vi "Autonomous Independent.vi"   [LabVIEW 2017]
doc: "This VI is called when autonomous begins, and will automatically be terminated when autonomous ends. You can carry out timed or sensor driven robot movement independently without needing to return to the caller."
uses:
  <vilib>/Rock Robotics/WPI/Solenoid/WPI_SolenoidValue.ctl
  <vilib>/Rock Robotics/WPI/ThirdParty/Phoenix-LabVIEW/Motor Controller/Controls/CTRE_Phoenix_MotorControl_ControlMode.ctl
  <vilib>/Rock Robotics/Network Tables/NT Read Number.vi
  <vilib>/Rock Robotics/WPI/Solenoid/WPI_SolenoidSetEnum.vi
  <vilib>/Rock Robotics/Network Tables/NT Write String.vi
panel:
  # "Be sure to right-click and choose Data Operations>>Make Current Value default if you want to save the array values with the VI"
types:
  T1 = enum16{"do_nothing", "cross_baseline_short", "cross_baseline_long", "hot_from_middle", "if_hot_2_cube_else_1_cube", "if_hot_1_cube_else_1_cube", "exchange_from_middle", "forward_switch_if_hot", "exchange_from_outside", "if_hot_2_cube_else_baseline", "if_hot_3_cube_else_baseline", "exchange_and_hot_switch", "hot_from_middle_diagonal", "yet to be named", "If_hot_1_else_baseline", "hot_2_from_middle", ""}
  T2 = typedef "WPI_SolenoidDevRef.ctl" = cluster{"DevStatus":errorcluster, "Pneumatics Control Module":u8, "Forward Solenoid Channel":T3, "Reverse Solenoid Channel":T3}
  T3 = typedef "WPI_SolenoidChannel.ctl" = enum8{"Solenoid 0", "Solenoid 1", "Solenoid 2", "Solenoid 3", "Solenoid 4", "Solenoid 5", "Solenoid 6", "Solenoid 7", "Invalid"}
  T4 = typedef "WPI_SolenoidValue.ctl" = enum16{"Off", "On", "Forward", "Reverse"}
  T5 = typedef "WPI_MotorControlDeviceRef.ctl" = cluster{"DeviceStatus":errorcluster, "Type":T6, "PWM":cluster{"PWM Channel":T7, "DeadBand":T8}, "CAN":cluster{"Device Number":u8, "SetOutput VI Ref":variant, "GetOutput VI Ref":variant, "Enable VI Ref":variant, "Disable VI Ref":variant, "Data":variant}, "Invert":bool, "DIO PWM":cluster{"PWM \"Enable\" Channel":T7, "DIOChannel":T9, "PWM Rate":dbl}}
  T6 = typedef "WPI_MotorControlType.ctl" = enum16{"PWM", "CAN", "DIO PWM"}
  T7 = typedef "FPGA_DIOPWMChannel.ctl" = enum8{"PWM 0", "PWM 1", "PWM 2", "PWM 3", "PWM 4", "PWM 5", "PWM 6", "PWM 7", "PWM 8", "PWM 9", "PWM MXP 0", "PWM MXP 1", "PWM MXP 2", "PWM MXP 3", "PWM MXP 4", "PWM MXP 5", "PWM MXP 6", "PWM MXP 7", "PWM MXP 8", "PWM MXP 9", "Invalid"}
  T8 = typedef "WPI_PWMDeadband.ctl" = cluster{"Name":string, "maxPositivePwm":i32, "minPositivePwm":i32, "centerPwm":i32, "maxNegativePwm":i32, "minNegativePwm":i32, "angularRange":u16}
  T9 = typedef "FPGA_DIOChannel.ctl" = enum8{"DIO 0", "DIO 1", "DIO 2", "DIO 3", "DIO 4", "DIO 5", "DIO 6", "DIO 7", "DIO 8", "DIO 9", "DIO MXP 0", "DIO MXP 1", "DIO MXP 2", "DIO MXP 3", "DIO MXP 4", "DIO MXP 5", "DIO MXP 6", "DIO MXP 7", "DIO MXP 8", "DIO MXP 9", "DIO MXP 10", "DIO MXP 11", "DIO MXP 12", "DIO MXP 13", "DIO MXP 14", "DIO MXP 15", "SPI Port CS1", "SPI Port CS2", "SPI Port CS3", "SPI Port MISO", "SPI Port MOSI", "Invalid"}
  T10 = typedef "CTRE_Phoenix_MotorControl_ControlMode.ctl" = u16
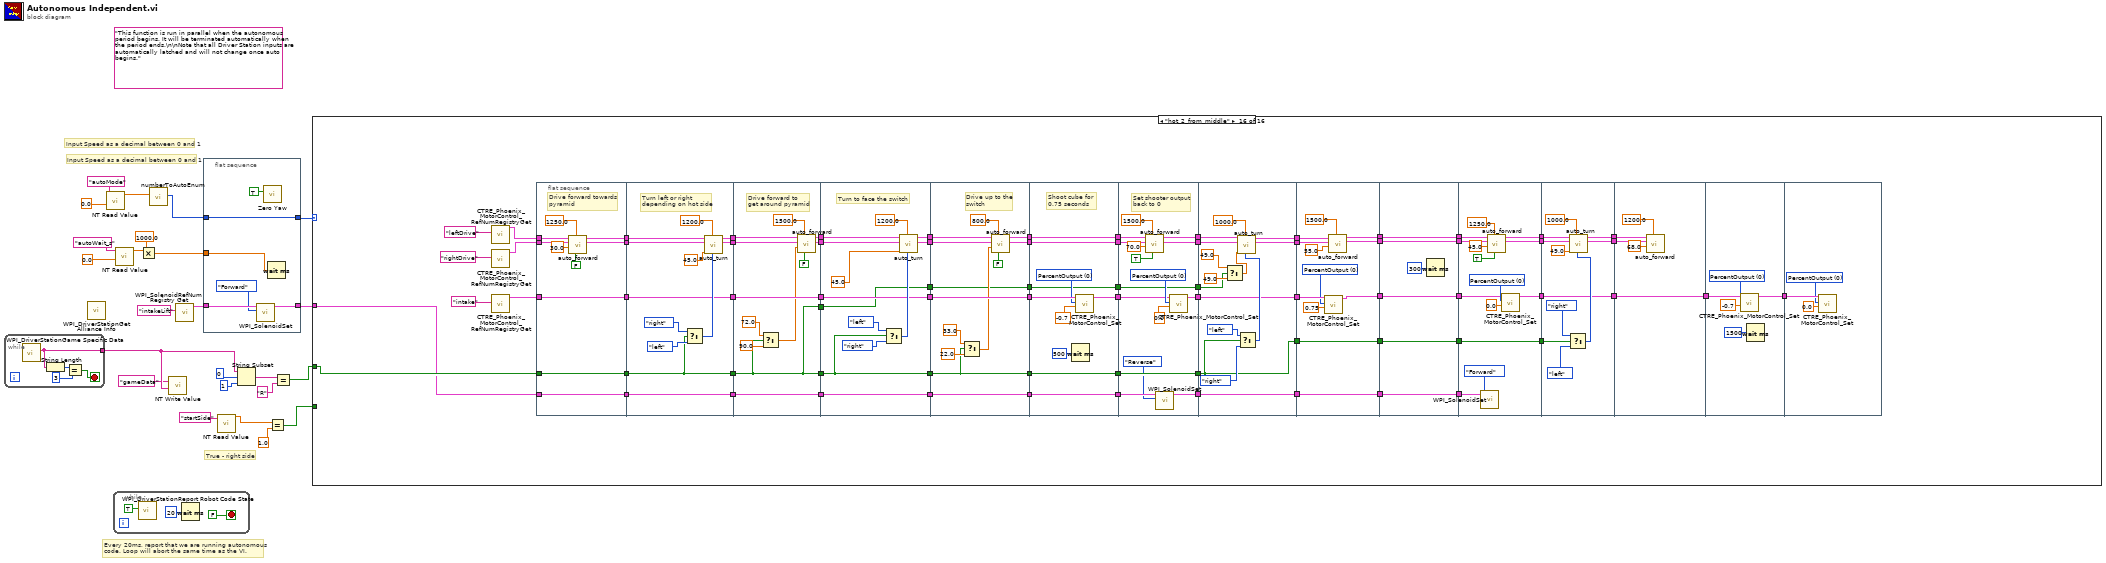
[diagram p0: block diagram]
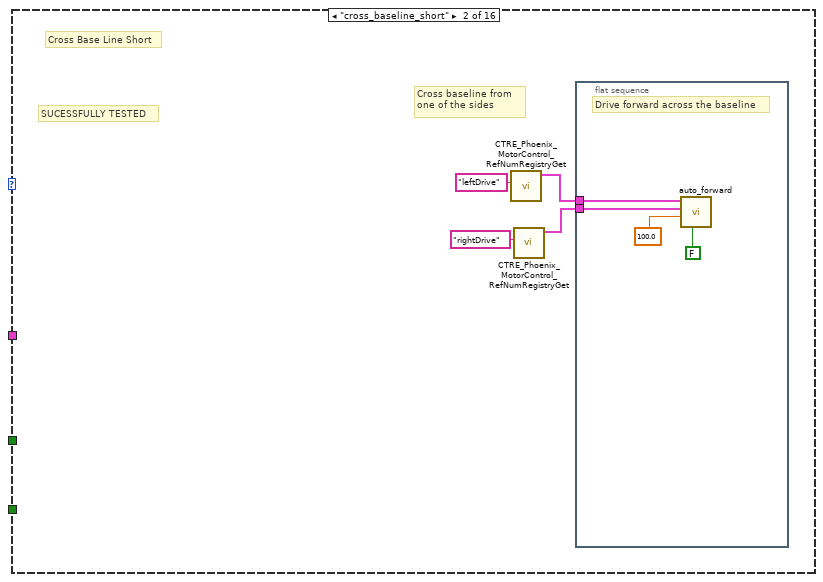
[diagram p3: hidden frame]
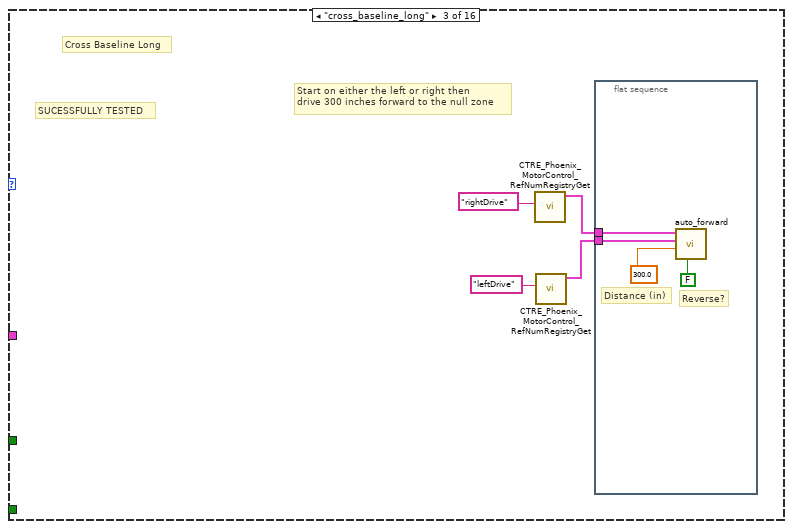
[diagram p4: hidden frame]
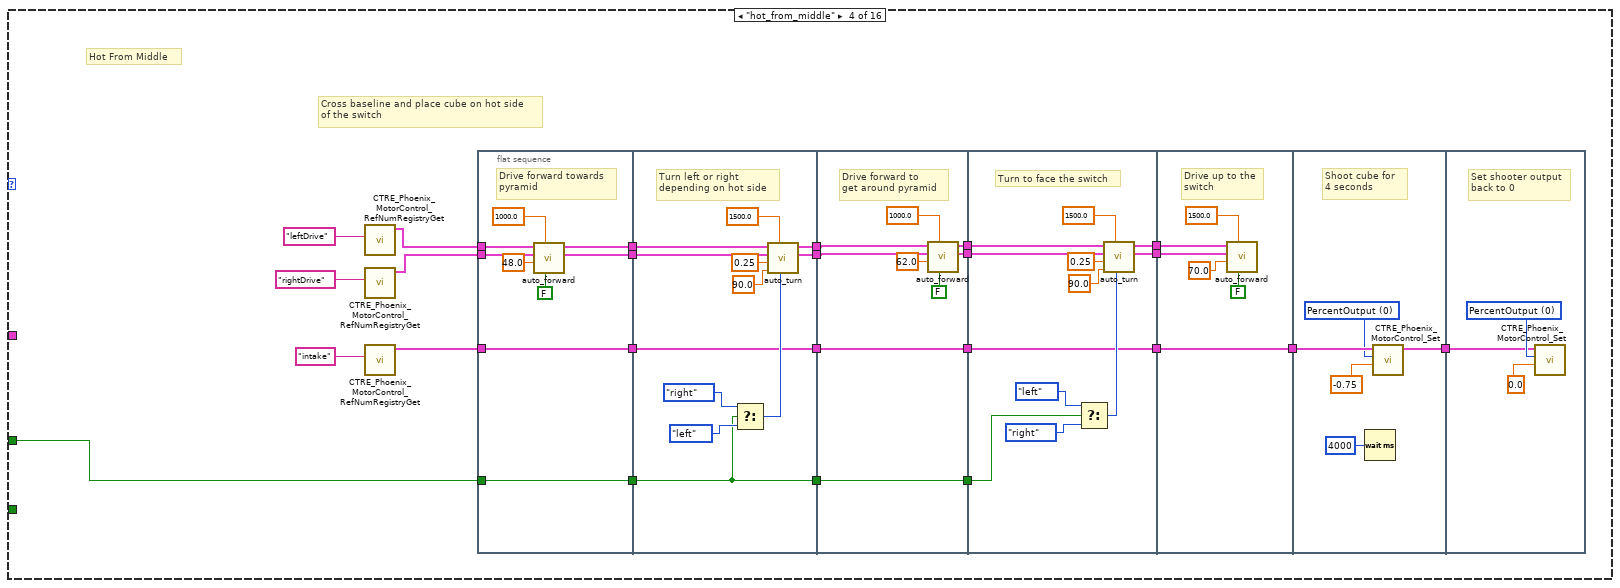
[diagram p5: hidden frame]
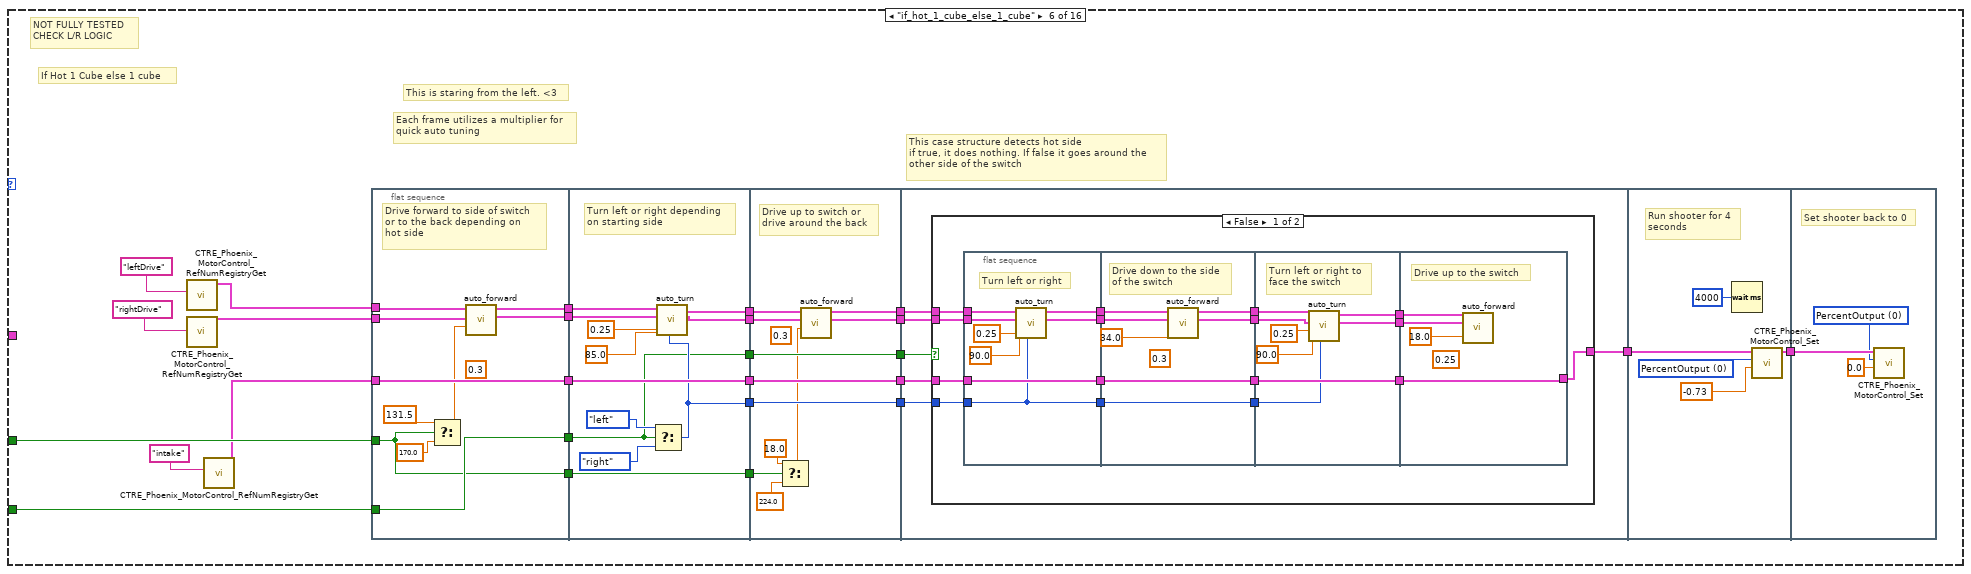
[diagram p7: hidden frame]
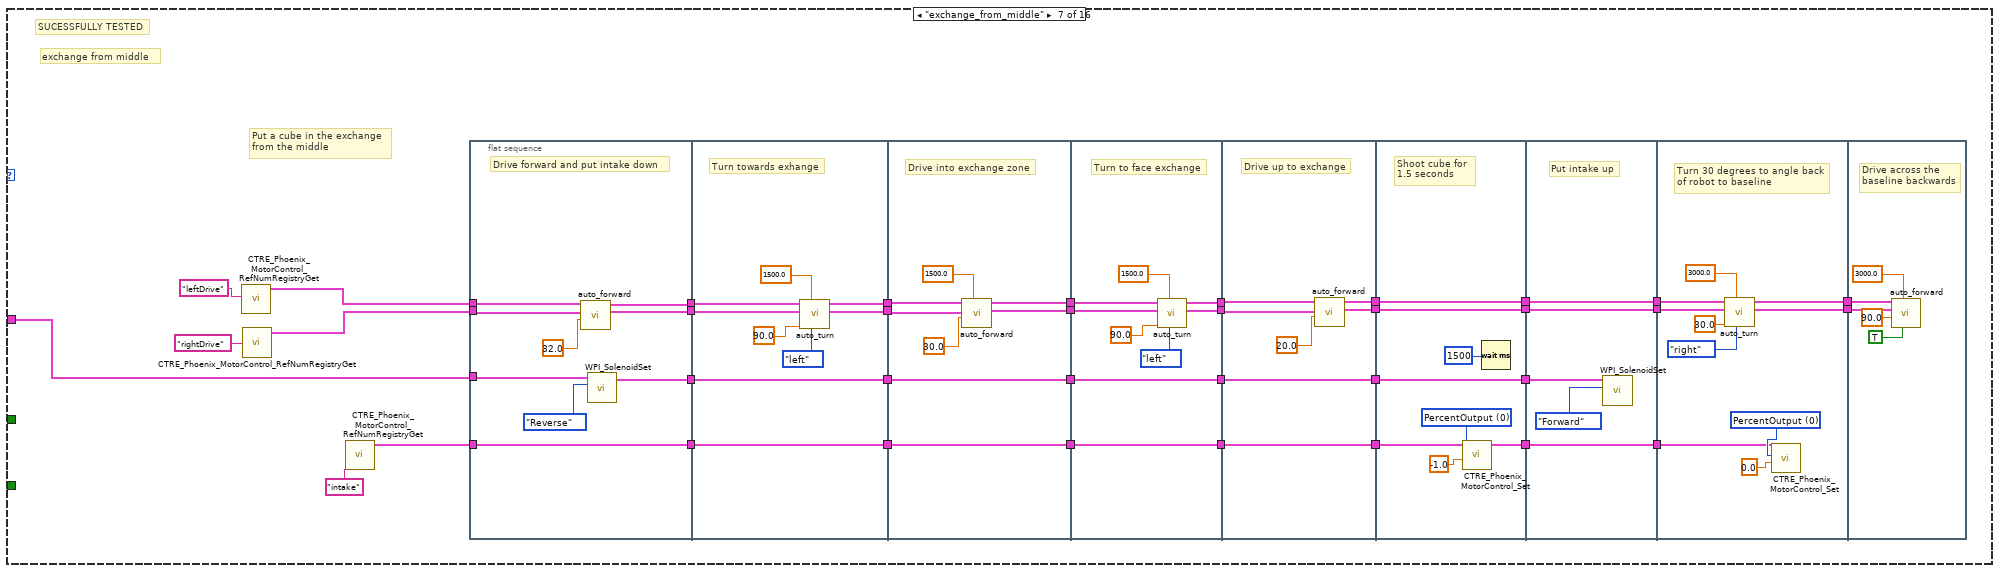
[diagram p9: hidden frame]
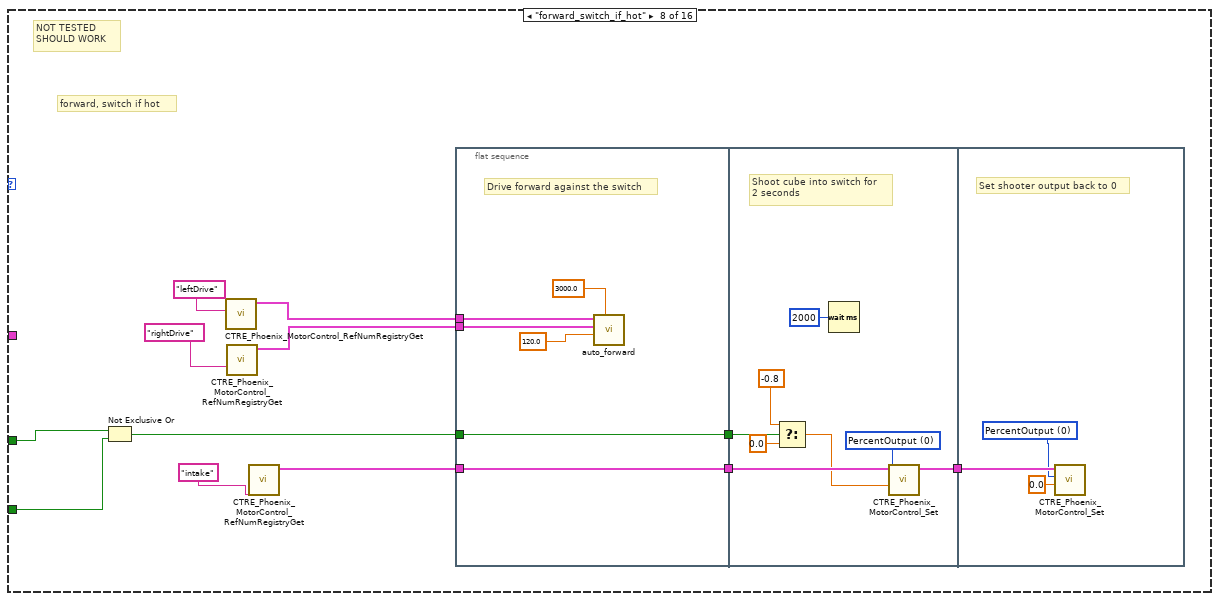
[diagram p10: hidden frame]
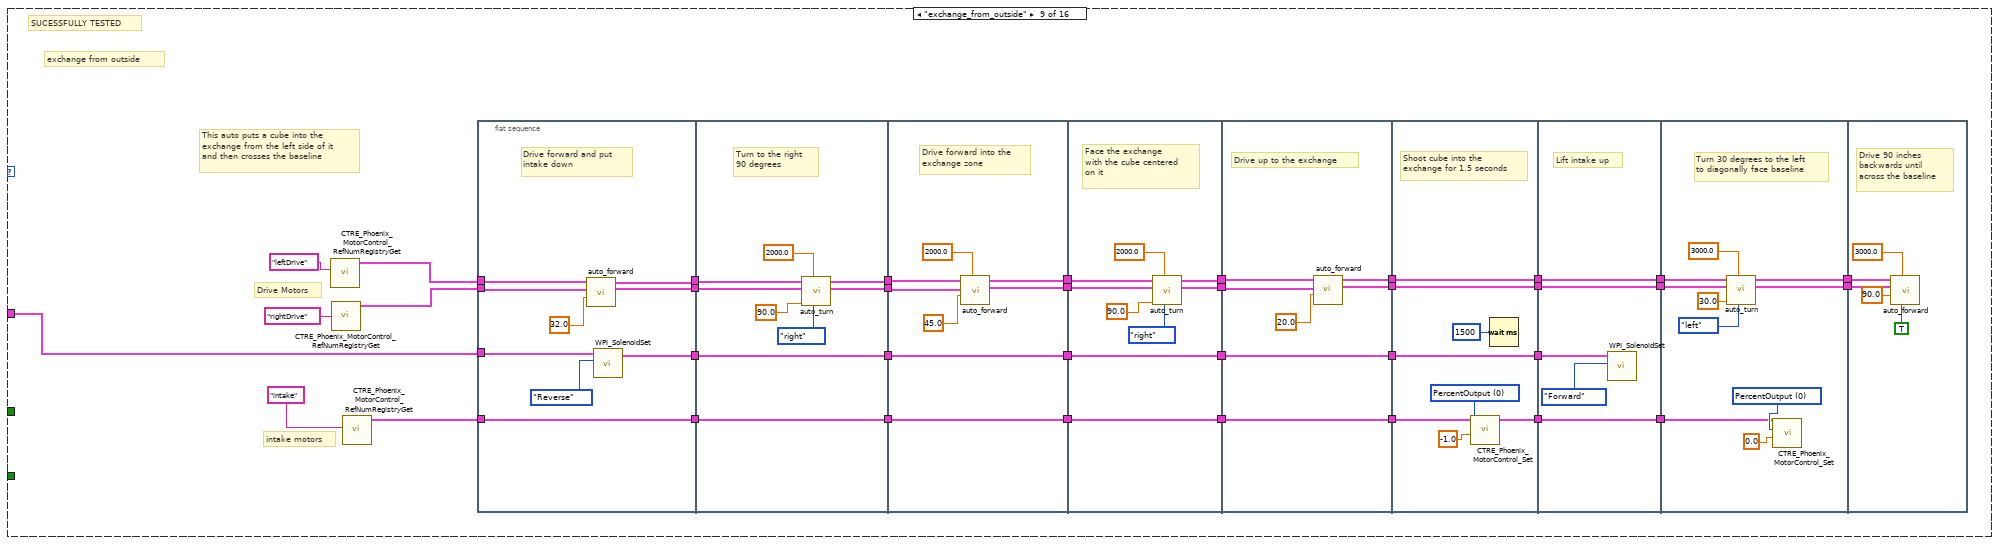
[diagram p11: hidden frame]
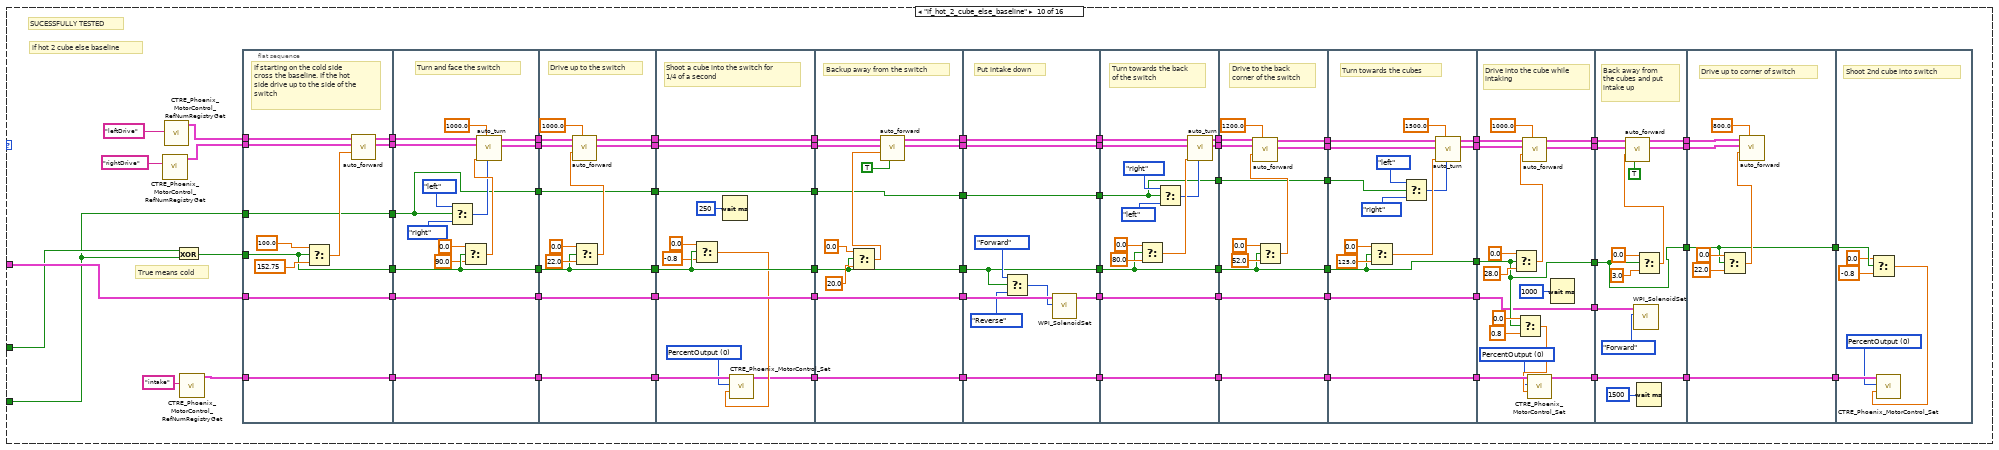
[diagram p12: hidden frame]
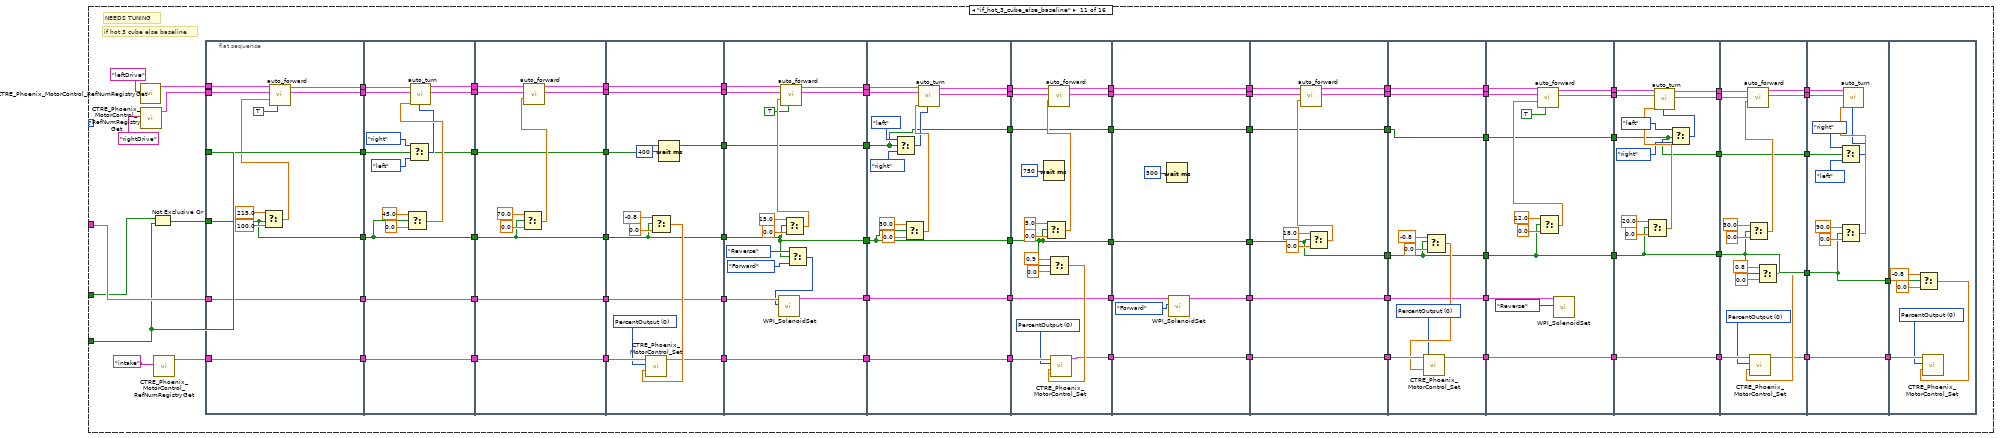
[diagram p13: hidden frame]
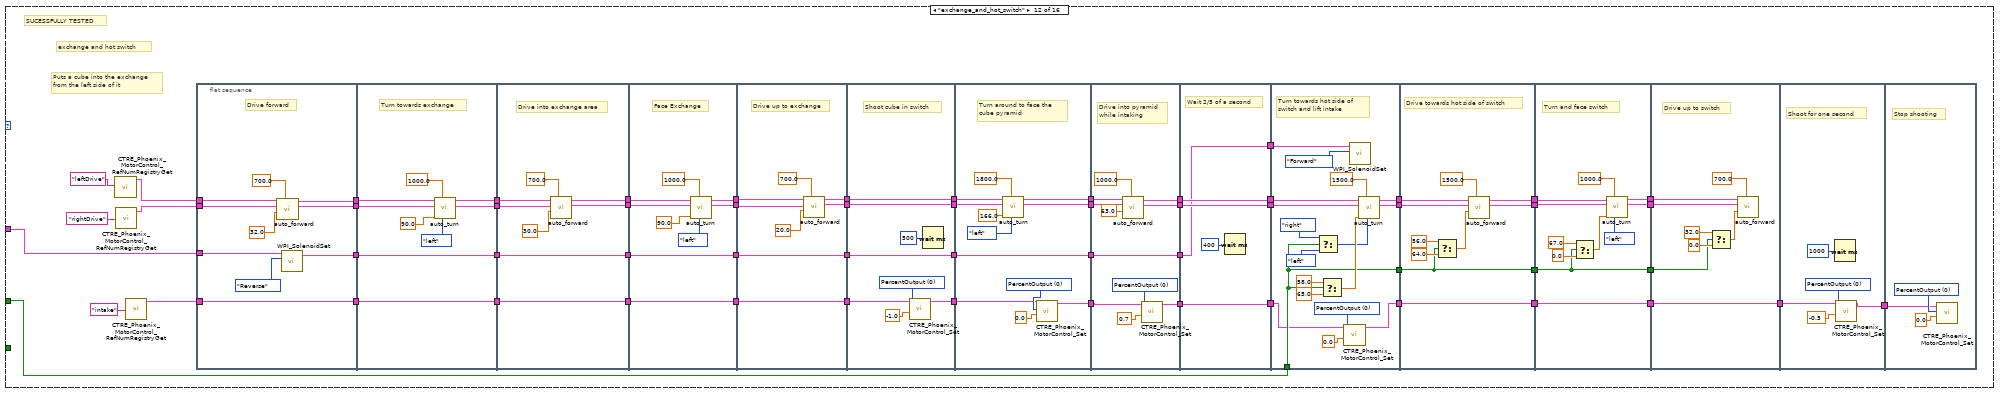
[diagram p14: hidden frame]
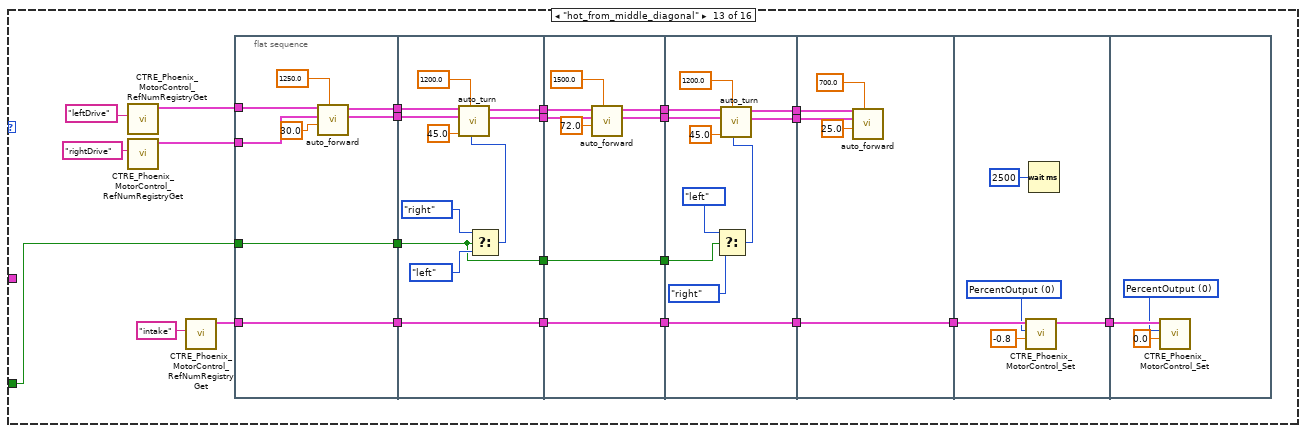
[diagram p15: hidden frame]
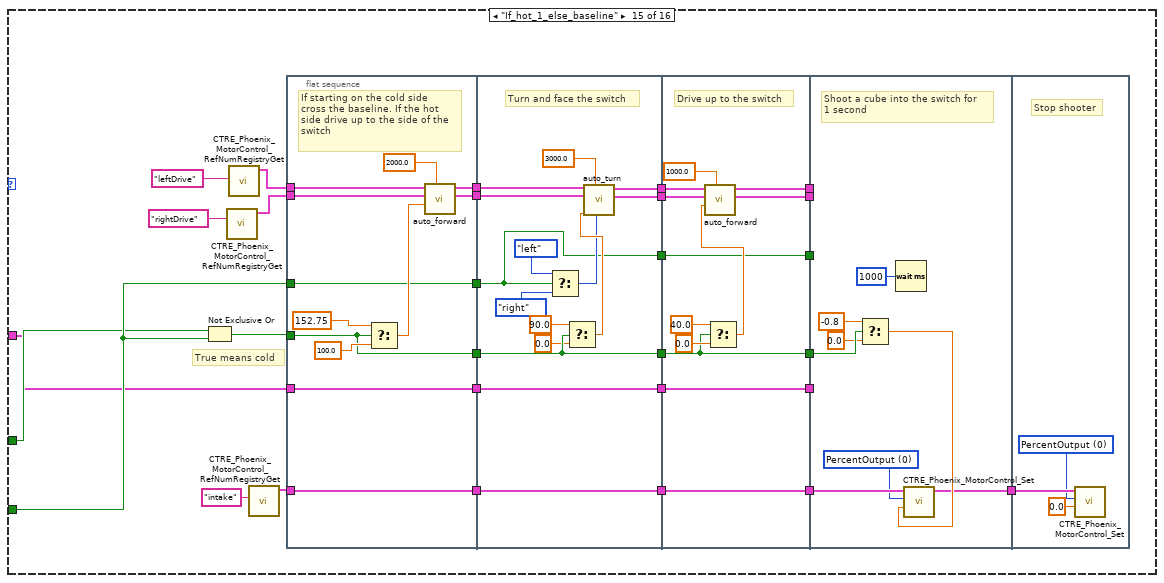
[diagram p17: hidden frame]
diagram:
  (unwired) "This function is run in parallel when the autonomous period begins. It will be terminated automatically when the period ends.\n\nNote that all Driver Station inputs are automatically latched and will not change once auto begins."
  # "True - right side"
  # "Input Speed as a decimal between 0 and 1"
  # "Input Speed as a decimal between 0 and 1"
  # "Every 20ms, report that we are running autonomous\ncode. Loop will abort the same time as the VI."
  n1 = while {
    tunnel: [w28] -> w2
    stop <- w25 stop-if-true
    n2 = call <vilib>:"WPI_DriverStationGame Specific Data.vi"() -> ("Game Specific Data"=w28:string)  [unwired: 11 in]
    n3 = String Length(string=w28) -> (length=w27:i32)
    n4 = Equal?(x=w27, y=3) -> (x = y?=w25:bool)
  }
  n5 = call <vilib>:"WPI_DriverStationGet Alliance Info.vi"() -> ()  [unwired: 12 out]
  n6 = call-poly <vilib>:"NT Read Value.vi"("Default Value"=0.0, "Name"="autoMode") -> ("Numeric"=w5:dbl)  [unwired: 8 in, 1 out]
  n7 = while {
    stop <- FALSE stop-if-true
    n8 = call <vilib>:"WPI_DriverStationReport Robot Code State.vi"("Autonomous"=TRUE) -> ()  [unwired: 10 in, 1 out]
    n9 = Wait (ms)(milliseconds to wait=u32 20) -> ()  [unwired: 1 out]
  }
  n10 = call-poly <vilib>:"NT Read Value.vi"("Default Value"=0.0, "Name"="autoWait_s") -> ("Numeric"=w23:dbl)  [unwired: 8 in, 1 out]
  n11 = Multiply(x=w23, y=1000.0) -> (x*y=w17:dbl)
  n12 = call "numberToAutoEnum.vi"("inNumber"=w5) -> ("outEnum"=w3:T1)  [unwired: 10 in]
  n13 = call-poly <vilib>:"NT Write Value.vi"("String"=w2, "Name"="gameData") -> ()  [unwired: 9 in, 1 out]
  n14 = call <vilib>:"WPI_SolenoidRefNum Registry Get.vi"("refnum name"="intakeLift") -> ("SolenoidDevRef"=w15:T2)  [unwired: 9 in, 1 out]
  n15 = flat-sequence {
    tunnel: w17 -> [w37]
    tunnel: w15 -> [w36]
    tunnel: [w34] -> w14
    tunnel: [w32] -> w4
    tunnel: w3 -> [w32]
    frame #0 {
      n16 = call-poly <vilib>:"WPI_SolenoidSet.vi"("Value"=WPI_SolenoidValue."Forward", "SolenoidDevRef"=w36) -> ("SolenoidDevRef"=w34:T2)  [unwired: 8 in, 1 out]
      n17 = call <vilib>:"Zero Yaw.vi"("Zero"=TRUE) -> ()  [unwired: 11 in]
      n18 = Wait (ms)(milliseconds to wait=w37) -> ()  [unwired: 1 out]
    }
  }
  n19 = call-poly <vilib>:"NT Read Value.vi"("Name"="startSide") -> ("Numeric"=w19:dbl)  [unwired: 9 in, 1 out]
  n20 = String Subset(string=w2, offset (0)=0, length (rest)=1 ("length (rest)")) -> (substring=w11:string)
  n21 = Equal?(x=w19, y=1.0) -> (x = y?=w13:bool)
  n22 = Equal?(x=w11, y="R") -> (x = y?=w9:bool)
  n23 = case shown="\"hot_2_from_middle\"" w4 {
    tunnel: w9 -> [_ _ _ w72 _ w152 _ w360 _ w496 w723 w1000 w1205 _ w1265 w1390]
    tunnel: w13 -> [_ _ _ _ _ w139 _ w359 _ w495 w724 _ _ _ w1266 _]
    tunnel: w14 -> [_ _ _ _ _ _ w263 _ w386 w561 w787 w1001 _ _ w1264 w1375]
    frame "do_nothing", Default {
      # "Do Nothing"
      # "Auto 0\nDefault Auto\nDo Nothing"
    }
    frame "cross_baseline_short" {
      # "Cross Base Line Short"
      # "Cross baseline from \none of the sides"
      # "SUCESSFULLY TESTED"
      n24 = call <vilib>:"CTRE_Phoenix_MotorControl_RefNumRegistryGet.vi"("refnum name"="leftDrive") -> ("PhoenixMotorControlDevRef"=w41:T5)  [unwired: 9 in, 1 out]
      n25 = call <vilib>:"CTRE_Phoenix_MotorControl_RefNumRegistryGet.vi"("refnum name"="rightDrive") -> ("PhoenixMotorControlDevRef"=w40:T5)  [unwired: 9 in, 1 out]
      n26 = flat-sequence {
        tunnel: w41 -> [w43]
        tunnel: w40 -> [w42]
        frame #0 {
          # "Drive forward across the baseline"
          n27 = call "auto_forward.vi"("reverse?"=FALSE, "distance (in)"=100.0, "rightDrive"=w42, "leftDrive"=w43) -> ()  [unwired: 6 in, 2 out]
        }
      }
    }
    frame "cross_baseline_long" {
      # "Cross Baseline Long"
      # "SUCESSFULLY TESTED"
      # "Start on either the left or right then \ndrive 300 inches forward to the null zone"
      n28 = call <vilib>:"CTRE_Phoenix_MotorControl_RefNumRegistryGet.vi"("refnum name"="rightDrive") -> ("PhoenixMotorControlDevRef"=w48:T5)  [unwired: 9 in, 1 out]
      n29 = call <vilib>:"CTRE_Phoenix_MotorControl_RefNumRegistryGet.vi"("refnum name"="leftDrive") -> ("PhoenixMotorControlDevRef"=w46:T5)  [unwired: 9 in, 1 out]
      n30 = flat-sequence {
        tunnel: w48 -> [w51]
        tunnel: w46 -> [w52]
        frame #0 {
          # "Reverse?"
          # "Distance (in)"
          n31 = call "auto_forward.vi"("reverse?"=FALSE, "distance (in)"=300.0, "rightDrive"=w52, "leftDrive"=w51) -> ()  [unwired: 6 in, 2 out]
        }
      }
    }
    frame "hot_from_middle" {
      # "Hot From Middle"
      # "Cross baseline and place cube on hot side\nof the switch"
      n32 = call <vilib>:"CTRE_Phoenix_MotorControl_RefNumRegistryGet.vi"("refnum name"="leftDrive") -> ("PhoenixMotorControlDevRef"=w74:T5)  [unwired: 9 in, 1 out]
      n33 = call <vilib>:"CTRE_Phoenix_MotorControl_RefNumRegistryGet.vi"("refnum name"="rightDrive") -> ("PhoenixMotorControlDevRef"=w73:T5)  [unwired: 9 in, 1 out]
      n34 = call <vilib>:"CTRE_Phoenix_MotorControl_RefNumRegistryGet.vi"("refnum name"="intake") -> ("PhoenixMotorControlDevRef"=w59:T5)  [unwired: 9 in, 1 out]
      n35 = flat-sequence {
        tunnel: w74 -> [w86]
        tunnel: w73 -> [w85]
        tunnel: [w83] -> w57
        tunnel: [w80] -> w56
        tunnel: w72 -> [w82]
        tunnel: [w82] -> w55
        tunnel: [w81] -> w54
        tunnel: w59 -> [w81]
        tunnel: w57 -> [w98]
        tunnel: w56 -> [w97]
        tunnel: w55 -> [w89]
        tunnel: [w91] -> w71
        tunnel: [w90] -> w70
        tunnel: [w89] -> w67
        tunnel: [w88] -> w60
        tunnel: w54 -> [w88]
        tunnel: w71 -> [w105]
        tunnel: w70 -> [w104]
        tunnel: [w103] -> w69
        tunnel: [w102] -> w68
        tunnel: w67 -> [w101]
        tunnel: [w101] -> w66
        tunnel: [w100] -> w61
        tunnel: w60 -> [w100]
        tunnel: w69 -> [w114]
        tunnel: w68 -> [w113]
        tunnel: w66 -> [w112]
        tunnel: [w111] -> w65
        tunnel: [w110] -> w64
        tunnel: [w109] -> w62
        tunnel: w61 -> [w109]
        tunnel: w65 -> [w123]
        tunnel: w64 -> [w122]
        tunnel: [w121] -> w63
        tunnel: w62 -> [w121]
        tunnel: w63 -> [w130]
        tunnel: [w127] -> w58
        tunnel: w58 -> [w131]
        frame #0 {
          # "Drive forward towards\npyramid"
          n36 = call "auto_forward.vi"("reverse?"=FALSE, "timeout (ms)"=1000.0, "distance (in)"=48.0, "rightDrive"=w85, "leftDrive"=w86) -> ("rightDrive"=w80:T5, "leftDrive"=w83:T5)  [unwired: 5 in]
        }
        frame #1 {
          # "Turn left or right \ndepending on hot side"
          n37 = Select(t=enum16{"right", "left"}."right" ("direction"), s=w89, f=enum16{"right", "left"}."left" ("direction")) -> (s? t:f=w92:enum16{"right", "left"})
          n38 = call "auto_turn.vi"("direction"=w92, "timeout (ms)"=1500.0, "angle"=90.0, "speed"=0.25, "rightDrive"=w97, "leftDrive"=w98) -> ("rightDrive"=w90:T5, "leftDrive"=w91:T5)  [unwired: 4 in]
        }
        frame #2 {
          # "Drive forward to\nget around pyramid"
          n39 = call "auto_forward.vi"("reverse?"=FALSE, "timeout (ms)"=1000.0, "distance (in)"=62.0, "rightDrive"=w104, "leftDrive"=w105) -> ("rightDrive"=w102:T5, "leftDrive"=w103:T5)  [unwired: 5 in]
        }
        frame #3 {
          # "Turn to face the switch"
          n40 = Select(t=enum16{"right", "left"}."left" ("direction"), s=w112, f=enum16{"right", "left"}."right" ("direction")) -> (s? t:f=w115:enum16{"right", "left"})
          n41 = call "auto_turn.vi"("direction"=w115, "timeout (ms)"=1500.0, "angle"=90.0, "speed"=0.25, "rightDrive"=w113, "leftDrive"=w114) -> ("rightDrive"=w110:T5, "leftDrive"=w111:T5)  [unwired: 4 in]
        }
        frame #4 {
          # "Drive up to the\nswitch"
          n42 = call "auto_forward.vi"("reverse?"=FALSE, "timeout (ms)"=1500.0, "distance (in)"=70.0, "rightDrive"=w122, "leftDrive"=w123) -> ()  [unwired: 5 in, 2 out]
        }
        frame #5 {
          w129 = T10 0 items=["PercentOutput"=0, "Position"=1, "Velocity"=2, "Current"=3, "Follower"=5, "MotionProfile"=6, "MotionMagic"=7, "MotionMagicArc"=8, "MotionProfileArc"=10, "Disabled"=15] ("Control Mode")
          # "Shoot cube for \n4 seconds"
          n43 = Wait (ms)(milliseconds to wait=u32 4000) -> ()  [unwired: 1 out]
          n44 = call <vilib>:"CTRE_Phoenix_MotorControl_Set.vi"("Output"=-0.75, "Control Mode"=w129, "PhoenixMotorControlDevRef"=w130) -> ("PhoenixMotorControlDevRef"=w127:T5)  [unwired: 7 in, 1 out]
        }
        frame #6 {
          w133 = T10 0 items=["PercentOutput"=0, "Position"=1, "Velocity"=2, "Current"=3, "Follower"=5, "MotionProfile"=6, "MotionMagic"=7, "MotionMagicArc"=8, "MotionProfileArc"=10, "Disabled"=15] ("Control Mode")
          # "Set shooter output\nback to 0"
          n45 = call <vilib>:"CTRE_Phoenix_MotorControl_Set.vi"("Output"=0.0, "Control Mode"=w133, "PhoenixMotorControlDevRef"=w131) -> ()  [unwired: 7 in, 2 out]
        }
      }
    }
    frame "if_hot_2_cube_else_1_cube" {
      # "If Hot 2 Cube else 1 Cube"
      # "NOT YET PROGRAMMED"
    }
    frame "if_hot_1_cube_else_1_cube" {
      # "If Hot 1 Cube else 1 cube"
      # "This case structure detects hot side\nif true, it does nothing. If false it goes around the\nother side of the switch"
      # "NOT FULLY TESTED\nCHECK L/R LOGIC"
      # "Each frame utilizes a multiplier for\nquick auto tuning"
      # "This is staring from the left. <3"
      n46 = call <vilib>:"CTRE_Phoenix_MotorControl_RefNumRegistryGet.vi"("refnum name"="leftDrive") -> ("PhoenixMotorControlDevRef"=w159:T5)  [unwired: 9 in, 1 out]
      n47 = call <vilib>:"CTRE_Phoenix_MotorControl_RefNumRegistryGet.vi"("refnum name"="rightDrive") -> ("PhoenixMotorControlDevRef"=w158:T5)  [unwired: 9 in, 1 out]
      n48 = call <vilib>:"CTRE_Phoenix_MotorControl_RefNumRegistryGet.vi"("refnum name"="intake") -> ("PhoenixMotorControlDevRef"=w145:T5)  [unwired: 9 in, 1 out]
      n49 = flat-sequence {
        tunnel: [w166] -> w156
        tunnel: [w165] -> w155
        tunnel: [w161] -> w151
        tunnel: [w163] -> w146
        tunnel: [w162] -> w140
        tunnel: w159 -> [w169]
        tunnel: w158 -> [w168]
        tunnel: w152 -> [w161]
        tunnel: w145 -> [w163]
        tunnel: w139 -> [w162]
        tunnel: w156 -> [w181]
        tunnel: w155 -> [w180]
        tunnel: [w178] -> w154
        tunnel: [w177] -> w153
        tunnel: w151 -> [w172]
        tunnel: [w172] -> w150
        tunnel: [w176] -> w147
        tunnel: w146 -> [w176]
        tunnel: w140 -> [w170]
        tunnel: [w173] -> w137
        tunnel: [w170] -> w135
        tunnel: w154 -> [w192]
        tunnel: w153 -> [w191]
        tunnel: w150 -> [w190]
        tunnel: [w188] -> w148
        tunnel: w147 -> [w188]
        tunnel: [w187] -> w144
        tunnel: [w186] -> w143
        tunnel: [w184] -> w138
        tunnel: w137 -> [w184]
        tunnel: [w183] -> w136
        tunnel: w135 -> [w183]
        tunnel: w148 -> [w198]
        tunnel: w144 -> [w197]
        tunnel: w143 -> [w196]
        tunnel: [w195] -> w141
        tunnel: w138 -> [w194]
        tunnel: w136 -> [w193]
        tunnel: w141 -> [w245]
        tunnel: [w243] -> w134
        tunnel: w134 -> [w250]
        frame #0 {
          (unwired) 0.3 ("speed (decimal)")
          # "Drive forward to side of switch\nor to the back depending on \nhot side"
          n50 = Select(t=131.5, s=w161, f=170.0) -> (s? t:f=w160:dbl)
          n51 = call "auto_forward.vi"("distance (in)"=w160, "rightDrive"=w168, "leftDrive"=w169) -> ("rightDrive"=w165:T5, "leftDrive"=w166:T5)  [unwired: 7 in]
        }
        frame #1 {
          # "Turn left or right depending\non starting side"
          n52 = Select(t=enum16{"right", "left"}."left" ("direction"), s=w170, f=enum16{"right", "left"}."right" ("direction")) -> (s? t:f=w173:enum16{"right", "left"})
          n53 = call "auto_turn.vi"("direction"=w173, "angle"=85.0, "speed"=0.25, "rightDrive"=w180, "leftDrive"=w181) -> ("rightDrive"=w177:T5, "leftDrive"=w178:T5)  [unwired: 5 in]
        }
        frame #2 {
          (unwired) 0.3 ("speed (decimal)")
          # "Drive up to switch or\ndrive around the back"
          n54 = Select(t=18.0, s=w190, f=224.0) -> (s? t:f=w182:dbl)
          n55 = call "auto_forward.vi"("distance (in)"=w182, "rightDrive"=w191, "leftDrive"=w192) -> ("rightDrive"=w186:T5, "leftDrive"=w187:T5)  [unwired: 7 in]
        }
        frame #3 {
          n56 = case shown="False" w193 {
            tunnel: w198 -> [w205 w242]
            tunnel: w197 -> [w214 _]
            tunnel: w196 -> [w213 _]
            tunnel: [w202 w242] -> w195
            tunnel: w194 -> [w201 _]
            frame False {
              n57 = flat-sequence {
                tunnel: w214 -> [w222]
                tunnel: w213 -> [w221]
                tunnel: [w219] -> w212
                tunnel: [w218] -> w211
                tunnel: [w217] -> w206
                tunnel: w205 -> [w217]
                tunnel: w201 -> [w216]
                tunnel: [w216] -> w199
                tunnel: w212 -> [w229]
                tunnel: w211 -> [w228]
                tunnel: [w227] -> w210
                tunnel: [w226] -> w209
                tunnel: w206 -> [w225]
                tunnel: [w225] -> w204
                tunnel: [w224] -> w200
                tunnel: w199 -> [w224]
                tunnel: w210 -> [w237]
                tunnel: w209 -> [w236]
                tunnel: [w234] -> w208
                tunnel: [w233] -> w207
                tunnel: w204 -> [w232]
                tunnel: [w232] -> w203
                tunnel: w200 -> [w231]
                tunnel: w208 -> [w241]
                tunnel: w207 -> [w240]
                tunnel: [w239] -> w202
                tunnel: w203 -> [w239]
                frame #0 {
                  # "Turn left or right"
                  n58 = call "auto_turn.vi"("direction"=w216, "angle"=90.0, "speed"=0.25, "rightDrive"=w221, "leftDrive"=w222) -> ("rightDrive"=w218:T5, "leftDrive"=w219:T5)  [unwired: 5 in]
                }
                frame #1 {
                  (unwired) 0.3 ("speed (decimal)")
                  # "Drive down to the side\nof the switch"
                  n59 = call "auto_forward.vi"("distance (in)"=34.0, "rightDrive"=w228, "leftDrive"=w229) -> ("rightDrive"=w226:T5, "leftDrive"=w227:T5)  [unwired: 7 in]
                }
                frame #2 {
                  # "Turn left or right to\nface the switch"
                  n60 = call "auto_turn.vi"("direction"=w231, "angle"=90.0, "speed"=0.25, "rightDrive"=w236, "leftDrive"=w237) -> ("rightDrive"=w233:T5, "leftDrive"=w234:T5)  [unwired: 5 in]
                }
                frame #3 {
                  (unwired) 0.25 ("speed (decimal)")
                  # "Drive up to the switch"
                  n61 = call "auto_forward.vi"("distance (in)"=18.0, "rightDrive"=w240, "leftDrive"=w241) -> ()  [unwired: 7 in, 2 out]
                }
              }
            }
            frame True {
            }
          }
        }
        frame #4 {
          w247 = T10 0 items=["PercentOutput"=0, "Position"=1, "Velocity"=2, "Current"=3, "Follower"=5, "MotionProfile"=6, "MotionMagic"=7, "MotionMagicArc"=8, "MotionProfileArc"=10, "Disabled"=15] ("Control Mode")
          # "Run shooter for 4\nseconds"
          n62 = Wait (ms)(milliseconds to wait=u32 4000) -> ()  [unwired: 1 out]
          n63 = call <vilib>:"CTRE_Phoenix_MotorControl_Set.vi"("Output"=-0.73, "Control Mode"=w247, "PhoenixMotorControlDevRef"=w245) -> ("PhoenixMotorControlDevRef"=w243:T5)  [unwired: 7 in, 1 out]
        }
        frame #5 {
          w248 = T10 0 items=["PercentOutput"=0, "Position"=1, "Velocity"=2, "Current"=3, "Follower"=5, "MotionProfile"=6, "MotionMagic"=7, "MotionMagicArc"=8, "MotionProfileArc"=10, "Disabled"=15] ("Control Mode")
          # "Set shooter back to 0"
          n64 = call <vilib>:"CTRE_Phoenix_MotorControl_Set.vi"("Output"=0.0, "Control Mode"=w248, "PhoenixMotorControlDevRef"=w250) -> ()  [unwired: 7 in, 2 out]
        }
      }
    }
    frame "exchange_from_middle" {
      # "exchange from middle"
      # "Put a cube in the exchange \nfrom the middle"
      # "SUCESSFULLY TESTED"
      n65 = call <vilib>:"CTRE_Phoenix_MotorControl_RefNumRegistryGet.vi"("refnum name"="leftDrive") -> ("PhoenixMotorControlDevRef"=w284:T5)  [unwired: 9 in, 1 out]
      n66 = call <vilib>:"CTRE_Phoenix_MotorControl_RefNumRegistryGet.vi"("refnum name"="rightDrive") -> ("PhoenixMotorControlDevRef"=w283:T5)  [unwired: 9 in, 1 out]
      n67 = call <vilib>:"CTRE_Phoenix_MotorControl_RefNumRegistryGet.vi"("refnum name"="intake") -> ("PhoenixMotorControlDevRef"=w278:T5)  [unwired: 9 in, 1 out]
      n68 = flat-sequence {
        tunnel: w283 -> [w294]
        tunnel: w284 -> [w295]
        tunnel: [w293] -> w282
        tunnel: [w292] -> w281
        tunnel: [w291] -> w279
        tunnel: w278 -> [w291]
        tunnel: w263 -> [w288]
        tunnel: [w287] -> w262
        tunnel: w282 -> [w304]
        tunnel: w281 -> [w303]
        tunnel: [w300] -> w277
        tunnel: w279 -> [w300]
        tunnel: [w299] -> w275
        tunnel: [w298] -> w274
        tunnel: w262 -> [w296]
        tunnel: [w296] -> w261
        tunnel: w277 -> [w312]
        tunnel: [w312] -> w276
        tunnel: w275 -> [w309]
        tunnel: w274 -> [w310]
        tunnel: [w308] -> w273
        tunnel: [w307] -> w272
        tunnel: w261 -> [w306]
        tunnel: [w306] -> w260
        tunnel: w276 -> [w321]
        tunnel: [w321] -> w271
        tunnel: w273 -> [w318]
        tunnel: w272 -> [w317]
        tunnel: [w316] -> w269
        tunnel: [w315] -> w268
        tunnel: w260 -> [w313]
        tunnel: [w313] -> w259
        tunnel: w271 -> [w328]
        tunnel: [w328] -> w270
        tunnel: w269 -> [w326]
        tunnel: w268 -> [w325]
        tunnel: [w324] -> w267
        tunnel: [w323] -> w266
        tunnel: w259 -> [w322]
        tunnel: [w322] -> w258
        tunnel: w270 -> [w336]
        tunnel: [w335] -> w253
        tunnel: [w331] -> w257
        tunnel: w267 -> [w331]
        tunnel: [w330] -> w255
        tunnel: w266 -> [w330]
        tunnel: w258 -> [w329]
        tunnel: [w329] -> w251
        tunnel: w257 -> [w341]
        tunnel: [w341] -> w256
        tunnel: w255 -> [w340]
        tunnel: [w340] -> w254
        tunnel: w253 -> [w339]
        tunnel: [w339] -> w252
        tunnel: w251 -> [w338]
        tunnel: w256 -> [w350]
        tunnel: w254 -> [w349]
        tunnel: [w348] -> w265
        tunnel: [w347] -> w264
        tunnel: w252 -> [w344]
        tunnel: w265 -> [w356]
        tunnel: w264 -> [w355]
        frame #0 {
          # "Drive forward and put intake down"
          n69 = call "auto_forward.vi"("distance (in)"=32.0 ("speed (decimal)"), "rightDrive"=w294, "leftDrive"=w295) -> ("rightDrive"=w292:T5, "leftDrive"=w293:T5)  [unwired: 7 in]
          n70 = call-poly <vilib>:"WPI_SolenoidSet.vi"("Value"=WPI_SolenoidValue."Reverse", "SolenoidDevRef"=w288) -> ("SolenoidDevRef"=w287:T2)  [unwired: 8 in, 1 out]
        }
        frame #1 {
          # "Turn towards exhange"
          n71 = call "auto_turn.vi"("direction"=enum16{"right", "left"}."left", "timeout (ms)"=1500.0, "angle"=90.0, "rightDrive"=w303, "leftDrive"=w304) -> ("rightDrive"=w298:T5, "leftDrive"=w299:T5)  [unwired: 5 in]
        }
        frame #2 {
          # "Drive into exchange zone"
          n72 = call "auto_forward.vi"("timeout (ms)"=1500.0, "distance (in)"=30.0 ("speed (decimal)"), "rightDrive"=w310, "leftDrive"=w309) -> ("rightDrive"=w307:T5, "leftDrive"=w308:T5)  [unwired: 6 in]
        }
        frame #3 {
          # "Turn to face exchange"
          n73 = call "auto_turn.vi"("direction"=enum16{"right", "left"}."left", "timeout (ms)"=1500.0, "angle"=90.0, "rightDrive"=w317, "leftDrive"=w318) -> ("rightDrive"=w315:T5, "leftDrive"=w316:T5)  [unwired: 5 in]
        }
        frame #4 {
          # "Drive up to exchange"
          n74 = call "auto_forward.vi"("distance (in)"=20.0 ("speed (decimal)"), "rightDrive"=w325, "leftDrive"=w326) -> ("rightDrive"=w323:T5, "leftDrive"=w324:T5)  [unwired: 7 in]
        }
        frame #5 {
          w332 = T10 0 items=["PercentOutput"=0, "Position"=1, "Velocity"=2, "Current"=3, "Follower"=5, "MotionProfile"=6, "MotionMagic"=7, "MotionMagicArc"=8, "MotionProfileArc"=10, "Disabled"=15] ("Control Mode")
          # "Shoot cube for \n1.5 seconds"
          n75 = call <vilib>:"CTRE_Phoenix_MotorControl_Set.vi"("Output"=-1.0, "Control Mode"=w332, "PhoenixMotorControlDevRef"=w336) -> ("PhoenixMotorControlDevRef"=w335:T5)  [unwired: 7 in, 1 out]
          n76 = Wait (ms)(milliseconds to wait=u32 1500) -> ()  [unwired: 1 out]
        }
        frame #6 {
          # "Put intake up"
          n77 = call-poly <vilib>:"WPI_SolenoidSet.vi"("Value"=WPI_SolenoidValue."Forward", "SolenoidDevRef"=w338) -> ()  [unwired: 8 in, 2 out]
        }
        frame #7 {
          w345 = T10 0 items=["PercentOutput"=0, "Position"=1, "Velocity"=2, "Current"=3, "Follower"=5, "MotionProfile"=6, "MotionMagic"=7, "MotionMagicArc"=8, "MotionProfileArc"=10, "Disabled"=15] ("Control Mode")
          # "Turn 30 degrees to angle back\nof robot to baseline"
          n78 = call "auto_turn.vi"("direction"=enum16{"right", "left"}."right", "timeout (ms)"=3000.0, "angle"=30.0, "rightDrive"=w349, "leftDrive"=w350) -> ("rightDrive"=w347:T5, "leftDrive"=w348:T5)  [unwired: 5 in]
          n79 = call <vilib>:"CTRE_Phoenix_MotorControl_Set.vi"("Output"=0.0, "Control Mode"=w345, "PhoenixMotorControlDevRef"=w344) -> ()  [unwired: 7 in, 2 out]
        }
        frame #8 {
          # "Drive across the\nbaseline backwards"
          n80 = call "auto_forward.vi"("reverse?"=TRUE, "timeout (ms)"=3000.0, "distance (in)"=90.0, "rightDrive"=w355, "leftDrive"=w356) -> ()  [unwired: 5 in, 2 out]
        }
      }
    }
    frame "forward_switch_if_hot" {
      # "forward, switch if hot"
      # "NOT TESTED\nSHOULD WORK"
      n81 = Not Exclusive Or(1:w359, 2:w360) -> (0:w357:bool)
      n82 = call <vilib>:"CTRE_Phoenix_MotorControl_RefNumRegistryGet.vi"("refnum name"="leftDrive") -> ("PhoenixMotorControlDevRef"=w367:T5)  [unwired: 9 in, 1 out]
      n83 = call <vilib>:"CTRE_Phoenix_MotorControl_RefNumRegistryGet.vi"("refnum name"="rightDrive") -> ("PhoenixMotorControlDevRef"=w366:T5)  [unwired: 9 in, 1 out]
      n84 = call <vilib>:"CTRE_Phoenix_MotorControl_RefNumRegistryGet.vi"("refnum name"="intake") -> ("PhoenixMotorControlDevRef"=w364:T5)  [unwired: 9 in, 1 out]
      n85 = flat-sequence {
        tunnel: w366 -> [w373]
        tunnel: w367 -> [w374]
        tunnel: [w371] -> w362
        tunnel: w364 -> [w371]
        tunnel: [w369] -> w358
        tunnel: w357 -> [w369]
        tunnel: w362 -> [w382]
        tunnel: [w381] -> w363
        tunnel: w358 -> [w378]
        tunnel: w363 -> [w384]
        frame #0 {
          # "Drive forward against the switch"
          n86 = call "auto_forward.vi"("timeout (ms)"=3000.0, "distance (in)"=120.0, "rightDrive"=w373, "leftDrive"=w374) -> ()  [unwired: 6 in, 2 out]
        }
        frame #1 {
          w380 = T10 0 items=["PercentOutput"=0, "Position"=1, "Velocity"=2, "Current"=3, "Follower"=5, "MotionProfile"=6, "MotionMagic"=7, "MotionMagicArc"=8, "MotionProfileArc"=10, "Disabled"=15] ("Control Mode")
          # "Shoot cube into switch for\n2 seconds"
          n87 = Select(t=-0.8, s=w378, f=0.0) -> (s? t:f=w375:dbl)
          n88 = Wait (ms)(milliseconds to wait=u32 2000) -> ()  [unwired: 1 out]
          n89 = call <vilib>:"CTRE_Phoenix_MotorControl_Set.vi"("Output"=w375, "Control Mode"=w380, "PhoenixMotorControlDevRef"=w382) -> ("PhoenixMotorControlDevRef"=w381:T5)  [unwired: 7 in, 1 out]
        }
        frame #2 {
          w383 = T10 0 items=["PercentOutput"=0, "Position"=1, "Velocity"=2, "Current"=3, "Follower"=5, "MotionProfile"=6, "MotionMagic"=7, "MotionMagicArc"=8, "MotionProfileArc"=10, "Disabled"=15] ("Control Mode")
          # "Set shooter output back to 0"
          n90 = call <vilib>:"CTRE_Phoenix_MotorControl_Set.vi"("Output"=0.0, "Control Mode"=w383, "PhoenixMotorControlDevRef"=w384) -> ()  [unwired: 7 in, 2 out]
        }
      }
    }
    frame "exchange_from_outside" {
      # "exchange from outside"
      # "SUCESSFULLY TESTED"
      # "intake motors"
      # "Drive Motors"
      # "This auto puts a cube into the\nexchange from the left side of it\nand then crosses the baseline"
      n91 = call <vilib>:"CTRE_Phoenix_MotorControl_RefNumRegistryGet.vi"("refnum name"="leftDrive") -> ("PhoenixMotorControlDevRef"=w390:T5)  [unwired: 9 in, 1 out]
      n92 = call <vilib>:"CTRE_Phoenix_MotorControl_RefNumRegistryGet.vi"("refnum name"="rightDrive") -> ("PhoenixMotorControlDevRef"=w389:T5)  [unwired: 9 in, 1 out]
      n93 = call <vilib>:"CTRE_Phoenix_MotorControl_RefNumRegistryGet.vi"("refnum name"="intake") -> ("PhoenixMotorControlDevRef"=w387:T5)  [unwired: 9 in, 1 out]
      n94 = flat-sequence {
        tunnel: w389 -> [w429]
        tunnel: w390 -> [w430]
        tunnel: [w428] -> w421
        tunnel: [w427] -> w420
        tunnel: [w426] -> w419
        tunnel: w387 -> [w426]
        tunnel: w386 -> [w423]
        tunnel: [w422] -> w418
        tunnel: w421 -> [w439]
        tunnel: w420 -> [w438]
        tunnel: [w435] -> w417
        tunnel: w419 -> [w435]
        tunnel: [w434] -> w416
        tunnel: [w433] -> w415
        tunnel: w418 -> [w431]
        tunnel: [w431] -> w414
        tunnel: w417 -> [w447]
        tunnel: [w447] -> w413
        tunnel: w416 -> [w444]
        tunnel: w415 -> [w445]
        tunnel: [w443] -> w412
        tunnel: [w442] -> w411
        tunnel: w414 -> [w441]
        tunnel: [w441] -> w410
        tunnel: w413 -> [w456]
        tunnel: [w456] -> w409
        tunnel: w412 -> [w453]
        tunnel: w411 -> [w452]
        tunnel: [w451] -> w408
        tunnel: [w450] -> w407
        tunnel: w410 -> [w448]
        tunnel: [w448] -> w406
        tunnel: w409 -> [w463]
        tunnel: [w463] -> w405
        tunnel: w408 -> [w461]
        tunnel: w407 -> [w460]
        tunnel: [w459] -> w404
        tunnel: [w458] -> w403
        tunnel: w406 -> [w457]
        tunnel: [w457] -> w402
        tunnel: w405 -> [w471]
        tunnel: [w470] -> w399
        tunnel: [w466] -> w401
        tunnel: w404 -> [w466]
        tunnel: [w465] -> w400
        tunnel: w403 -> [w465]
        tunnel: w402 -> [w464]
        tunnel: [w464] -> w398
        tunnel: w401 -> [w476]
        tunnel: [w476] -> w397
        tunnel: w400 -> [w475]
        tunnel: [w475] -> w396
        tunnel: w399 -> [w474]
        tunnel: [w474] -> w395
        tunnel: w398 -> [w473]
        tunnel: w397 -> [w485]
        tunnel: w396 -> [w484]
        tunnel: [w483] -> w394
        tunnel: [w482] -> w393
        tunnel: w395 -> [w479]
        tunnel: w394 -> [w491]
        tunnel: w393 -> [w490]
        frame #0 {
          # "Drive forward and put\nintake down"
          n95 = call "auto_forward.vi"("distance (in)"=32.0 ("speed (decimal)"), "rightDrive"=w429, "leftDrive"=w430) -> ("rightDrive"=w427:T5, "leftDrive"=w428:T5)  [unwired: 7 in]
          n96 = call-poly <vilib>:"WPI_SolenoidSet.vi"("Value"=WPI_SolenoidValue."Reverse", "SolenoidDevRef"=w423) -> ("SolenoidDevRef"=w422:T2)  [unwired: 8 in, 1 out]
        }
        frame #1 {
          # "Turn to the right\n90 degrees"
          n97 = call "auto_turn.vi"("direction"=enum16{"right", "left"}."right", "timeout (ms)"=2000.0, "angle"=90.0, "rightDrive"=w438, "leftDrive"=w439) -> ("rightDrive"=w433:T5, "leftDrive"=w434:T5)  [unwired: 5 in]
        }
        frame #2 {
          # "Drive forward into the\nexchange zone"
          n98 = call "auto_forward.vi"("timeout (ms)"=2000.0, "distance (in)"=45.0 ("speed (decimal)"), "rightDrive"=w445, "leftDrive"=w444) -> ("rightDrive"=w442:T5, "leftDrive"=w443:T5)  [unwired: 6 in]
        }
        frame #3 {
          # "Face the exchange\nwith the cube centered\non it"
          n99 = call "auto_turn.vi"("direction"=enum16{"right", "left"}."right", "timeout (ms)"=2000.0, "angle"=90.0, "rightDrive"=w452, "leftDrive"=w453) -> ("rightDrive"=w450:T5, "leftDrive"=w451:T5)  [unwired: 5 in]
        }
        frame #4 {
          # "Drive up to the exchange"
          n100 = call "auto_forward.vi"("distance (in)"=20.0 ("speed (decimal)"), "rightDrive"=w460, "leftDrive"=w461) -> ("rightDrive"=w458:T5, "leftDrive"=w459:T5)  [unwired: 7 in]
        }
        frame #5 {
          w467 = T10 0 items=["PercentOutput"=0, "Position"=1, "Velocity"=2, "Current"=3, "Follower"=5, "MotionProfile"=6, "MotionMagic"=7, "MotionMagicArc"=8, "MotionProfileArc"=10, "Disabled"=15] ("Control Mode")
          # "Shoot cube into the\nexchange for 1.5 seconds"
          n101 = call <vilib>:"CTRE_Phoenix_MotorControl_Set.vi"("Output"=-1.0, "Control Mode"=w467, "PhoenixMotorControlDevRef"=w471) -> ("PhoenixMotorControlDevRef"=w470:T5)  [unwired: 7 in, 1 out]
          n102 = Wait (ms)(milliseconds to wait=u32 1500) -> ()  [unwired: 1 out]
        }
        frame #6 {
          # "Lift intake up"
          n103 = call-poly <vilib>:"WPI_SolenoidSet.vi"("Value"=WPI_SolenoidValue."Forward", "SolenoidDevRef"=w473) -> ()  [unwired: 8 in, 2 out]
        }
        frame #7 {
          w480 = T10 0 items=["PercentOutput"=0, "Position"=1, "Velocity"=2, "Current"=3, "Follower"=5, "MotionProfile"=6, "MotionMagic"=7, "MotionMagicArc"=8, "MotionProfileArc"=10, "Disabled"=15] ("Control Mode")
          # "Turn 30 degrees to the left\nto diagonally face baseline"
          n104 = call "auto_turn.vi"("direction"=enum16{"right", "left"}."left", "timeout (ms)"=3000.0, "angle"=30.0, "rightDrive"=w484, "leftDrive"=w485) -> ("rightDrive"=w482:T5, "leftDrive"=w483:T5)  [unwired: 5 in]
          n105 = call <vilib>:"CTRE_Phoenix_MotorControl_Set.vi"("Output"=0.0, "Control Mode"=w480, "PhoenixMotorControlDevRef"=w479) -> ()  [unwired: 7 in, 2 out]
        }
        frame #8 {
          # "Drive 90 inches\nbackwards until \nacross the baseline"
          n106 = call "auto_forward.vi"("reverse?"=TRUE, "timeout (ms)"=3000.0, "distance (in)"=90.0, "rightDrive"=w490, "leftDrive"=w491) -> ()  [unwired: 5 in, 2 out]
        }
      }
    }
    frame "if_hot_2_cube_else_baseline" {
      # "if hot 2 cube else baseline"
      # "SUCESSFULLY TESTED"
      # "True means cold"
      n107 = call <vilib>:"CTRE_Phoenix_MotorControl_RefNumRegistryGet.vi"("refnum name"="rightDrive") -> ("PhoenixMotorControlDevRef"=w564:T5)  [unwired: 9 in, 1 out]
      n108 = call <vilib>:"CTRE_Phoenix_MotorControl_RefNumRegistryGet.vi"("refnum name"="leftDrive") -> ("PhoenixMotorControlDevRef"=w565:T5)  [unwired: 9 in, 1 out]
      n109 = Exclusive Or(1:w495, 2:w496) -> (0:w494:bool)
      n110 = call <vilib>:"CTRE_Phoenix_MotorControl_RefNumRegistryGet.vi"("refnum name"="intake") -> ("PhoenixMotorControlDevRef"=w563:T5)  [unwired: 9 in, 1 out]
      n111 = flat-sequence {
        tunnel: w565 -> [w573]
        tunnel: w564 -> [w572]
        tunnel: w494 -> [w569]
        tunnel: [w571] -> w560
        tunnel: [w570] -> w559
        tunnel: [w569] -> w558
        tunnel: w563 -> [w568]
        tunnel: [w568] -> w557
        tunnel: [w567] -> w556
        tunnel: w561 -> [w567]
        tunnel: [w566] -> w508
        tunnel: w495 -> [w566]
        tunnel: w560 -> [w591]
        tunnel: w559 -> [w590]
        tunnel: w558 -> [w589]
        tunnel: [w589] -> w555
        tunnel: [w585] -> w554
        tunnel: [w584] -> w553
        tunnel: w557 -> [w583]
        tunnel: [w583] -> w552
        tunnel: w556 -> [w582]
        tunnel: [w582] -> w551
        tunnel: w508 -> [w577]
        tunnel: [w577] -> w503
        tunnel: w555 -> [w595]
        tunnel: w554 -> [w600]
        tunnel: w553 -> [w599]
        tunnel: w552 -> [w598]
        tunnel: [w598] -> w550
        tunnel: [w597] -> w549
        tunnel: [w596] -> w548
        tunnel: [w595] -> w547
        tunnel: [w594] -> w546
        tunnel: w551 -> [w594]
        tunnel: [w592] -> w504
        tunnel: w503 -> [w592]
        tunnel: w550 -> [w615]
        tunnel: [w612] -> w545
        tunnel: w549 -> [w612]
        tunnel: [w611] -> w544
        tunnel: w548 -> [w611]
        tunnel: w547 -> [w610]
        tunnel: [w610] -> w543
        tunnel: [w609] -> w542
        tunnel: w546 -> [w609]
        tunnel: [w605] -> w541
        tunnel: [w604] -> w505
        tunnel: w504 -> [w604]
        tunnel: w545 -> [w627]
        tunnel: w544 -> [w626]
        tunnel: w543 -> [w619]
        tunnel: [w621] -> w540
        tunnel: [w620] -> w539
        tunnel: [w619] -> w538
        tunnel: [w618] -> w537
        tunnel: w542 -> [w618]
        tunnel: [w617] -> w536
        tunnel: w541 -> [w617]
        tunnel: [w616] -> w506
        tunnel: w505 -> [w616]
        tunnel: w540 -> [w637]
        tunnel: [w637] -> w535
        tunnel: w539 -> [w636]
        tunnel: [w636] -> w534
        tunnel: w538 -> [w630]
        tunnel: [w630] -> w533
        tunnel: w537 -> [w635]
        tunnel: [w634] -> w532
        tunnel: w536 -> [w634]
        tunnel: [w629] -> w509
        tunnel: [w628] -> w507
        tunnel: w506 -> [w628]
        tunnel: w535 -> [w651]
        tunnel: w534 -> [w650]
        tunnel: w533 -> [w644]
        tunnel: [w646] -> w531
        tunnel: [w645] -> w530
        tunnel: [w644] -> w529
        tunnel: [w643] -> w528
        tunnel: w532 -> [w643]
        tunnel: [w642] -> w510
        tunnel: w509 -> [w642]
        tunnel: w507 -> [w638]
        tunnel: [w638] -> w501
        tunnel: w531 -> [w661]
        tunnel: w530 -> [w660]
        tunnel: [w658] -> w527
        tunnel: [w657] -> w526
        tunnel: w529 -> [w656]
        tunnel: [w656] -> w525
        tunnel: [w655] -> w524
        tunnel: w528 -> [w655]
        tunnel: [w654] -> w511
        tunnel: w510 -> [w654]
        tunnel: [w652] -> w502
        tunnel: w501 -> [w652]
        tunnel: w527 -> [w678]
        tunnel: w526 -> [w677]
        tunnel: w525 -> [w671]
        tunnel: [w673] -> w523
        tunnel: [w672] -> w522
        tunnel: [w671] -> w521
        tunnel: [w670] -> w520
        tunnel: w524 -> [w670]
        tunnel: [w669] -> w512
        tunnel: w511 -> [w669]
        tunnel: w502 -> [w665]
        tunnel: w523 -> [w695]
        tunnel: w522 -> [w694]
        tunnel: w521 -> [w683]
        tunnel: w520 -> [w690]
        tunnel: [w685] -> w519
        tunnel: [w684] -> w518
        tunnel: [w683] -> w517
        tunnel: [w681] -> w516
        tunnel: [w680] -> w513
        tunnel: w512 -> [w680]
        tunnel: w519 -> [w704]
        tunnel: w518 -> [w703]
        tunnel: w517 -> [w696]
        tunnel: [w702] -> w500
        tunnel: [w708] -> w499
        tunnel: w516 -> [w708]
        tunnel: w513 -> [w707]
        tunnel: [w701] -> w498
        tunnel: [w696] -> w497
        tunnel: w500 -> [w716]
        tunnel: [w711] -> w515
        tunnel: w499 -> [w711]
        tunnel: [w710] -> w514
        tunnel: w498 -> [w715]
        tunnel: w497 -> [w710]
        tunnel: w515 -> [w722]
        tunnel: w514 -> [w720]
        frame #0 {
          # "If starting on the cold side\ncross the baseline. If the hot\nside drive up to the side of the\nswitch"
          n112 = Select(t=100.0, s=w569, f=152.75) -> (s? t:f=w574:dbl)
          n113 = call "auto_forward.vi"("distance (in)"=w574, "rightDrive"=w572, "leftDrive"=w573) -> ("rightDrive"=w570:T5, "leftDrive"=w571:T5)  [unwired: 7 in]
        }
        frame #1 {
          # "Turn and face the switch"
          n114 = Select(t=enum16{"right", "left"}."left" ("direction"), s=w577, f=enum16{"right", "left"}."right" ("direction")) -> (s? t:f=w580:enum16{"right", "left"})
          n115 = Select(t=0.0, s=w589, f=90.0) -> (s? t:f=w586:dbl)
          n116 = call "auto_turn.vi"("direction"=w580, "timeout (ms)"=1000.0, "angle"=w586, "rightDrive"=w590, "leftDrive"=w591) -> ("rightDrive"=w584:T5, "leftDrive"=w585:T5)  [unwired: 5 in]
        }
        frame #2 {
          # "Drive up to the switch"
          n117 = Select(t=0.0, s=w595, f=22.0) -> (s? t:f=w601:dbl)
          n118 = call "auto_forward.vi"("timeout (ms)"=1000.0, "distance (in)"=w601, "rightDrive"=w599, "leftDrive"=w600) -> ("rightDrive"=w596:T5, "leftDrive"=w597:T5)  [unwired: 6 in]
        }
        frame #3 {
          w614 = T10 0 items=["PercentOutput"=0, "Position"=1, "Velocity"=2, "Current"=3, "Follower"=5, "MotionProfile"=6, "MotionMagic"=7, "MotionMagicArc"=8, "MotionProfileArc"=10, "Disabled"=15] ("Control Mode")
          # "Shoot a cube into the switch for\n1/4 of a second"
          n119 = Select(t=0.0, s=w610, f=-0.8) -> (s? t:f=w606:dbl)
          n120 = Wait (ms)(milliseconds to wait=u32 250) -> ()  [unwired: 1 out]
          n121 = call <vilib>:"CTRE_Phoenix_MotorControl_Set.vi"("Output"=w606, "Control Mode"=w614, "PhoenixMotorControlDevRef"=w615) -> ("PhoenixMotorControlDevRef"=w605:T5)  [unwired: 7 in, 1 out]
        }
        frame #4 {
          # "Backup away from the switch"
          n122 = Select(t=0.0, s=w619, f=20.0 ("distance (in)")) -> (s? t:f=w622:dbl)
          n123 = call "auto_forward.vi"("reverse?"=TRUE, "distance (in)"=w622, "rightDrive"=w626, "leftDrive"=w627) -> ("rightDrive"=w620:T5, "leftDrive"=w621:T5)  [unwired: 6 in]
        }
        frame #5 {
          # "Put intake down"
          n124 = Select(t=WPI_SolenoidValue."Forward" ("Value"), s=w630, f=WPI_SolenoidValue."Reverse" ("Value")) -> (s? t:f=w633:T4)
          n125 = call-poly <vilib>:"WPI_SolenoidSet.vi"("Value"=w633, "SolenoidDevRef"=w635) -> ("SolenoidDevRef"=w629:T2)  [unwired: 8 in, 1 out]
        }
        frame #6 {
          # "Turn towards the back\nof the switch"
          n126 = Select(t=0.0, s=w644, f=80.0) -> (s? t:f=w647:dbl)
          n127 = Select(t=enum16{"right", "left"}."right" ("direction"), s=w638, f=enum16{"right", "left"}."left" ("direction")) -> (s? t:f=w639:enum16{"right", "left"})
          n128 = call "auto_turn.vi"("direction"=w639, "angle"=w647, "rightDrive"=w650, "leftDrive"=w651) -> ("rightDrive"=w645:T5, "leftDrive"=w646:T5)  [unwired: 6 in]
        }
        frame #7 {
          # "Drive to the back\ncorner of the switch"
          n129 = Select(t=0.0, s=w656, f=52.0) -> (s? t:f=w659:dbl)
          n130 = call "auto_forward.vi"("timeout (ms)"=1200.0, "distance (in)"=w659, "rightDrive"=w660, "leftDrive"=w661) -> ("rightDrive"=w657:T5, "leftDrive"=w658:T5)  [unwired: 6 in]
        }
        frame #8 {
          # "Turn towards the cubes"
          n131 = Select(t=0.0, s=w671, f=125.0) -> (s? t:f=w674:dbl)
          n132 = Select(t=enum16{"right", "left"}."left" ("direction"), s=w665, f=enum16{"right", "left"}."right" ("direction")) -> (s? t:f=w664:enum16{"right", "left"})
          n133 = call "auto_turn.vi"("direction"=w664, "timeout (ms)"=1500.0, "angle"=w674, "rightDrive"=w677, "leftDrive"=w678) -> ("rightDrive"=w672:T5, "leftDrive"=w673:T5)  [unwired: 5 in]
        }
        frame #9 {
          w682 = T10 0 items=["PercentOutput"=0, "Position"=1, "Velocity"=2, "Current"=3, "Follower"=5, "MotionProfile"=6, "MotionMagic"=7, "MotionMagicArc"=8, "MotionProfileArc"=10, "Disabled"=15] ("Control Mode")
          # "Drive into the cube while\nintaking"
          n134 = Select(t=0.0, s=w683, f=28.0) -> (s? t:f=w691:dbl)
          n135 = Select(t=0.0, s=w683, f=0.8) -> (s? t:f=w687:dbl)
          n136 = call "auto_forward.vi"("timeout (ms)"=1000.0, "distance (in)"=w691, "rightDrive"=w694, "leftDrive"=w695) -> ("rightDrive"=w684:T5, "leftDrive"=w685:T5)  [unwired: 6 in]
          n137 = call <vilib>:"CTRE_Phoenix_MotorControl_Set.vi"("Output"=w687, "Control Mode"=w682, "PhoenixMotorControlDevRef"=w690) -> ("PhoenixMotorControlDevRef"=w681:T5)  [unwired: 7 in, 1 out]
          n138 = Wait (ms)(milliseconds to wait=u32 1000) -> ()  [unwired: 1 out]
        }
        frame #10 {
          # "Back away from\nthe cubes and put\nintake up"
          n139 = call-poly <vilib>:"WPI_SolenoidSet.vi"("Value"=WPI_SolenoidValue."Forward", "SolenoidDevRef"=w707) -> ()  [unwired: 8 in, 2 out]
          n140 = Select(t=0.0, s=w696, f=3.0) -> (s? t:f=w697:dbl)
          n141 = call "auto_forward.vi"("reverse?"=TRUE, "distance (in)"=w697, "rightDrive"=w703, "leftDrive"=w704) -> ("rightDrive"=w701:T5, "leftDrive"=w702:T5)  [unwired: 6 in]
          n142 = Wait (ms)(milliseconds to wait=u32 1500) -> ()  [unwired: 1 out]
        }
        frame #11 {
          # "Drive up to corner of switch"
          n143 = Select(t=0.0, s=w710, f=22.0) -> (s? t:f=w712:dbl)
          n144 = call "auto_forward.vi"("timeout (ms)"=800.0, "distance (in)"=w712, "rightDrive"=w715, "leftDrive"=w716) -> ()  [unwired: 6 in, 2 out]
        }
        frame #12 {
          w721 = T10 0 items=["PercentOutput"=0, "Position"=1, "Velocity"=2, "Current"=3, "Follower"=5, "MotionProfile"=6, "MotionMagic"=7, "MotionMagicArc"=8, "MotionProfileArc"=10, "Disabled"=15] ("Control Mode")
          # "Shoot 2nd cube into switch"
          n145 = Select(t=0.0, s=w720, f=-0.8) -> (s? t:f=w717:dbl)
          n146 = call <vilib>:"CTRE_Phoenix_MotorControl_Set.vi"("Output"=w717, "Control Mode"=w721, "PhoenixMotorControlDevRef"=w722) -> ()  [unwired: 7 in, 2 out]
        }
      }
    }
    frame "if_hot_3_cube_else_baseline" {
      # "if hot 3 cube else baseline"
      # "NEEDS TUNING"
      n147 = call <vilib>:"CTRE_Phoenix_MotorControl_RefNumRegistryGet.vi"("refnum name"="leftDrive") -> ("PhoenixMotorControlDevRef"=w809:T5)  [unwired: 9 in, 1 out]
      n148 = call <vilib>:"CTRE_Phoenix_MotorControl_RefNumRegistryGet.vi"("refnum name"="rightDrive") -> ("PhoenixMotorControlDevRef"=w808:T5)  [unwired: 9 in, 1 out]
      n149 = Not Exclusive Or(1:w724, 2:w723) -> (0:w725:bool)
      n150 = call <vilib>:"CTRE_Phoenix_MotorControl_RefNumRegistryGet.vi"("refnum name"="intake") -> ("PhoenixMotorControlDevRef"=w797:T5)  [unwired: 9 in, 1 out]
      n151 = flat-sequence {
        tunnel: w809 -> [w821]
        tunnel: w808 -> [w820]
        tunnel: [w818] -> w805
        tunnel: [w817] -> w804
        tunnel: w725 -> [w814]
        tunnel: w724 -> [w815]
        tunnel: [w815] -> w803
        tunnel: [w814] -> w802
        tunnel: [w811] -> w798
        tunnel: w797 -> [w811]
        tunnel: w787 -> [w810]
        tunnel: [w810] -> w783
        tunnel: w805 -> [w835]
        tunnel: w804 -> [w834]
        tunnel: w803 -> [w822]
        tunnel: w802 -> [w825]
        tunnel: [w827] -> w801
        tunnel: [w826] -> w800
        tunnel: [w825] -> w799
        tunnel: w798 -> [w824]
        tunnel: [w824] -> w795
        tunnel: [w823] -> w784
        tunnel: w783 -> [w823]
        tunnel: [w822] -> w776
        tunnel: w801 -> [w846]
        tunnel: w800 -> [w845]
        tunnel: w799 -> [w840]
        tunnel: [w841] -> w796
        tunnel: w795 -> [w841]
        tunnel: [w840] -> w793
        tunnel: [w839] -> w791
        tunnel: [w838] -> w789
        tunnel: [w837] -> w785
        tunnel: w784 -> [w837]
        tunnel: [w836] -> w777
        tunnel: w776 -> [w836]
        tunnel: w796 -> [w858]
        tunnel: w793 -> [w850]
        tunnel: [w852] -> w792
        tunnel: w791 -> [w852]
        tunnel: [w851] -> w790
        tunnel: w789 -> [w851]
        tunnel: [w850] -> w788
        tunnel: [w849] -> w786
        tunnel: w785 -> [w849]
        tunnel: [w848] -> w778
        tunnel: w777 -> [w848]
        tunnel: [w847] -> w770
        tunnel: w792 -> [w874]
        tunnel: w790 -> [w873]
        tunnel: w788 -> [w862]
        tunnel: w786 -> [w870]
        tunnel: [w864] -> w782
        tunnel: [w863] -> w781
        tunnel: [w862] -> w780
        tunnel: [w861] -> w779
        tunnel: w778 -> [w861]
        tunnel: [w860] -> w771
        tunnel: w770 -> [w860]
        tunnel: [w859] -> w767
        tunnel: w782 -> [w888]
        tunnel: w781 -> [w887]
        tunnel: w780 -> [w878]
        tunnel: w779 -> [w875]
        tunnel: [w880] -> w775
        tunnel: [w879] -> w774
        tunnel: [w878] -> w773
        tunnel: [w877] -> w772
        tunnel: w771 -> [w877]
        tunnel: [w876] -> w768
        tunnel: w767 -> [w876]
        tunnel: [w875] -> w739
        tunnel: w775 -> [w905]
        tunnel: w774 -> [w904]
        tunnel: w773 -> [w891]
        tunnel: w772 -> [w900]
        tunnel: [w894] -> w769
        tunnel: w768 -> [w894]
        tunnel: [w893] -> w765
        tunnel: [w892] -> w763
        tunnel: [w891] -> w761
        tunnel: [w890] -> w758
        tunnel: w739 -> [w889]
        tunnel: [w889] -> w736
        tunnel: w769 -> [w914]
        tunnel: [w911] -> w766
        tunnel: w765 -> [w911]
        tunnel: [w910] -> w764
        tunnel: w763 -> [w910]
        tunnel: [w909] -> w762
        tunnel: w761 -> [w909]
        tunnel: [w908] -> w759
        tunnel: w758 -> [w908]
        tunnel: [w907] -> w749
        tunnel: [w906] -> w737
        tunnel: w736 -> [w906]
        tunnel: w766 -> [w925]
        tunnel: w764 -> [w924]
        tunnel: w762 -> [w919]
        tunnel: [w920] -> w760
        tunnel: w759 -> [w920]
        tunnel: [w919] -> w757
        tunnel: [w918] -> w755
        tunnel: [w917] -> w753
        tunnel: [w916] -> w750
        tunnel: w749 -> [w916]
        tunnel: [w915] -> w738
        tunnel: w737 -> [w915]
        tunnel: w760 -> [w936]
        tunnel: w757 -> [w929]
        tunnel: [w931] -> w756
        tunnel: w755 -> [w931]
        tunnel: [w930] -> w754
        tunnel: w753 -> [w930]
        tunnel: [w929] -> w752
        tunnel: [w928] -> w751
        tunnel: w750 -> [w928]
        tunnel: w738 -> [w927]
        tunnel: [w927] -> w734
        tunnel: [w926] -> w729
        tunnel: w756 -> [w949]
        tunnel: w754 -> [w948]
        tunnel: w752 -> [w939]
        tunnel: w751 -> [w944]
        tunnel: [w941] -> w748
        tunnel: [w940] -> w747
        tunnel: [w939] -> w746
        tunnel: [w938] -> w735
        tunnel: w734 -> [w938]
        tunnel: [w937] -> w730
        tunnel: w729 -> [w937]
        tunnel: w748 -> [w962]
        tunnel: w747 -> [w961]
        tunnel: w746 -> [w955]
        tunnel: [w957] -> w745
        tunnel: [w956] -> w744
        tunnel: [w955] -> w743
        tunnel: w735 -> [w951]
        tunnel: [w951] -> w732
        tunnel: [w950] -> w731
        tunnel: w730 -> [w950]
        tunnel: w745 -> [w977]
        tunnel: w744 -> [w976]
        tunnel: w743 -> [w968]
        tunnel: [w972] -> w742
        tunnel: [w971] -> w741
        tunnel: [w968] -> w740
        tunnel: [w970] -> w733
        tunnel: w732 -> [w970]
        tunnel: w731 -> [w969]
        tunnel: [w963] -> w727
        tunnel: w742 -> [w988]
        tunnel: w741 -> [w987]
        tunnel: w740 -> [w978]
        tunnel: w733 -> [w980]
        tunnel: [w979] -> w728
        tunnel: w727 -> [w979]
        tunnel: [w978] -> w726
        tunnel: w728 -> [w994]
        tunnel: w726 -> [w992]
        frame #0 {
          n152 = Select(t=215.0, s=w814, f=100.0) -> (s? t:f=w812:dbl)
          n153 = call "auto_forward.vi"("reverse?"=TRUE, "distance (in)"=w812, "rightDrive"=w820, "leftDrive"=w821) -> ("rightDrive"=w817:T5, "leftDrive"=w818:T5)  [unwired: 6 in]
        }
        frame #1 {
          n154 = Select(t=45.0, s=w825, f=0.0) -> (s? t:f=w831:dbl)
          n155 = Select(t=enum16{"right", "left"}."right" ("direction"), s=w822, f=enum16{"right", "left"}."left" ("direction")) -> (s? t:f=w828:enum16{"right", "left"})
          n156 = call "auto_turn.vi"("direction"=w828, "angle"=w831, "rightDrive"=w834, "leftDrive"=w835) -> ("rightDrive"=w826:T5, "leftDrive"=w827:T5)  [unwired: 6 in]
        }
        frame #2 {
          n157 = Select(t=70.0, s=w840, f=0.0) -> (s? t:f=w842:dbl)
          n158 = call "auto_forward.vi"("distance (in)"=w842, "rightDrive"=w845, "leftDrive"=w846) -> ("rightDrive"=w838:T5, "leftDrive"=w839:T5)  [unwired: 7 in]
        }
        frame #3 {
          w857 = T10 0 items=["PercentOutput"=0, "Position"=1, "Velocity"=2, "Current"=3, "Follower"=5, "MotionProfile"=6, "MotionMagic"=7, "MotionMagicArc"=8, "MotionProfileArc"=10, "Disabled"=15] ("Control Mode")
          n159 = Select(t=-0.8, s=w850, f=0.0) -> (s? t:f=w854:dbl)
          n160 = call <vilib>:"CTRE_Phoenix_MotorControl_Set.vi"("Output"=w854, "Control Mode"=w857, "PhoenixMotorControlDevRef"=w858) -> ("PhoenixMotorControlDevRef"=w847:T5)  [unwired: 7 in, 1 out]
          n161 = Wait (ms)(milliseconds to wait=u32 400) -> ()  [unwired: 1 out]
        }
        frame #4 {
          n162 = Select(t=15.0, s=w862, f=0.0) -> (s? t:f=w866:dbl)
          n163 = call "auto_forward.vi"("reverse?"=TRUE, "distance (in)"=w866, "rightDrive"=w873, "leftDrive"=w874) -> ("rightDrive"=w863:T5, "leftDrive"=w864:T5)  [unwired: 6 in]
          n164 = Select(t=WPI_SolenoidValue."Reverse" ("Value"), s=w862, f=WPI_SolenoidValue."Forward" ("Value")) -> (s? t:f=w867:T4)
          n165 = call-poly <vilib>:"WPI_SolenoidSet.vi"("Value"=w867, "SolenoidDevRef"=w870) -> ("SolenoidDevRef"=w859:T2)  [unwired: 8 in, 1 out]
        }
        frame #5 {
          n166 = Select(t=enum16{"right", "left"}."left" ("direction"), s=w875, f=enum16{"right", "left"}."right" ("direction")) -> (s? t:f=w881:enum16{"right", "left"})
          n167 = Select(t=30.0, s=w878, f=0.0) -> (s? t:f=w884:dbl)
          n168 = call "auto_turn.vi"("direction"=w881, "angle"=w884, "rightDrive"=w887, "leftDrive"=w888) -> ("rightDrive"=w879:T5, "leftDrive"=w880:T5)  [unwired: 6 in]
        }
        frame #6 {
          w899 = T10 0 items=["PercentOutput"=0, "Position"=1, "Velocity"=2, "Current"=3, "Follower"=5, "MotionProfile"=6, "MotionMagic"=7, "MotionMagicArc"=8, "MotionProfileArc"=10, "Disabled"=15] ("Control Mode")
          n169 = Wait (ms)(milliseconds to wait=u32 750) -> ()  [unwired: 1 out]
          n170 = Select(t=5.0, s=w891, f=0.0) -> (s? t:f=w901:dbl)
          n171 = call "auto_forward.vi"("distance (in)"=w901, "rightDrive"=w904, "leftDrive"=w905) -> ("rightDrive"=w892:T5, "leftDrive"=w893:T5)  [unwired: 7 in]
          n172 = Select(t=0.9, s=w891, f=0.0) -> (s? t:f=w896:dbl)
          n173 = call <vilib>:"CTRE_Phoenix_MotorControl_Set.vi"("Output"=w896, "Control Mode"=w899, "PhoenixMotorControlDevRef"=w900) -> ("PhoenixMotorControlDevRef"=w890:T5)  [unwired: 7 in, 1 out]
        }
        frame #7 {
          n174 = Wait (ms)(milliseconds to wait=u32 500) -> ()  [unwired: 1 out]
          n175 = call-poly <vilib>:"WPI_SolenoidSet.vi"("Value"=WPI_SolenoidValue."Forward", "SolenoidDevRef"=w914) -> ("SolenoidDevRef"=w907:T2)  [unwired: 8 in, 1 out]
        }
        frame #8 {
          n176 = Select(t=18.0, s=w919, f=0.0) -> (s? t:f=w921:dbl)
          n177 = call "auto_forward.vi"("distance (in)"=w921, "rightDrive"=w924, "leftDrive"=w925) -> ("rightDrive"=w917:T5, "leftDrive"=w918:T5)  [unwired: 7 in]
        }
        frame #9 {
          w932 = T10 0 items=["PercentOutput"=0, "Position"=1, "Velocity"=2, "Current"=3, "Follower"=5, "MotionProfile"=6, "MotionMagic"=7, "MotionMagicArc"=8, "MotionProfileArc"=10, "Disabled"=15] ("Control Mode")
          n178 = Select(t=-0.8, s=w929, f=0.0) -> (s? t:f=w933:dbl)
          n179 = call <vilib>:"CTRE_Phoenix_MotorControl_Set.vi"("Output"=w933, "Control Mode"=w932, "PhoenixMotorControlDevRef"=w936) -> ("PhoenixMotorControlDevRef"=w926:T5)  [unwired: 7 in, 1 out]
        }
        frame #10 {
          n180 = Select(t=12.0, s=w939, f=0.0) -> (s? t:f=w942:dbl)
          n181 = call "auto_forward.vi"("reverse?"=TRUE, "distance (in)"=w942, "rightDrive"=w948, "leftDrive"=w949) -> ("rightDrive"=w940:T5, "leftDrive"=w941:T5)  [unwired: 6 in]
          n182 = call-poly <vilib>:"WPI_SolenoidSet.vi"("Value"=WPI_SolenoidValue."Reverse", "SolenoidDevRef"=w944) -> ()  [unwired: 8 in, 2 out]
        }
        frame #11 {
          n183 = Select(t=20.0, s=w955, f=0.0) -> (s? t:f=w958:dbl)
          n184 = Select(t=enum16{"right", "left"}."left" ("direction"), s=w951, f=enum16{"right", "left"}."right" ("direction")) -> (s? t:f=w952:enum16{"right", "left"})
          n185 = call "auto_turn.vi"("direction"=w952, "angle"=w958, "rightDrive"=w961, "leftDrive"=w962) -> ("rightDrive"=w956:T5, "leftDrive"=w957:T5)  [unwired: 6 in]
        }
        frame #12 {
          w964 = T10 0 items=["PercentOutput"=0, "Position"=1, "Velocity"=2, "Current"=3, "Follower"=5, "MotionProfile"=6, "MotionMagic"=7, "MotionMagicArc"=8, "MotionProfileArc"=10, "Disabled"=15] ("Control Mode")
          n186 = Select(t=30.0, s=w968, f=0.0) -> (s? t:f=w973:dbl)
          n187 = call "auto_forward.vi"("distance (in)"=w973, "rightDrive"=w976, "leftDrive"=w977) -> ("rightDrive"=w971:T5, "leftDrive"=w972:T5)  [unwired: 7 in]
          n188 = Select(t=0.8, s=w968, f=0.0) -> (s? t:f=w965:dbl)
          n189 = call <vilib>:"CTRE_Phoenix_MotorControl_Set.vi"("Output"=w965, "Control Mode"=w964, "PhoenixMotorControlDevRef"=w969) -> ("PhoenixMotorControlDevRef"=w963:T5)  [unwired: 7 in, 1 out]
        }
        frame #13 {
          n190 = Select(t=enum16{"right", "left"}."right" ("direction"), s=w980, f=enum16{"right", "left"}."left" ("direction")) -> (s? t:f=w981:enum16{"right", "left"})
          n191 = Select(t=90.0, s=w978, f=0.0) -> (s? t:f=w984:dbl)
          n192 = call "auto_turn.vi"("direction"=w981, "angle"=w984, "rightDrive"=w987, "leftDrive"=w988) -> ()  [unwired: 6 in, 2 out]
        }
        frame #14 {
          w993 = T10 0 items=["PercentOutput"=0, "Position"=1, "Velocity"=2, "Current"=3, "Follower"=5, "MotionProfile"=6, "MotionMagic"=7, "MotionMagicArc"=8, "MotionProfileArc"=10, "Disabled"=15] ("Control Mode")
          n193 = Select(t=-0.8, s=w992, f=0.0) -> (s? t:f=w989:dbl)
          n194 = call <vilib>:"CTRE_Phoenix_MotorControl_Set.vi"("Output"=w989, "Control Mode"=w993, "PhoenixMotorControlDevRef"=w994) -> ()  [unwired: 7 in, 2 out]
        }
      }
    }
    frame "exchange_and_hot_switch" {
      # "exchange and hot switch"
      # "Puts a cube into the exchange\nfrom the left side of it"
      # "SUCESSFULLY TESTED"
      n195 = call <vilib>:"CTRE_Phoenix_MotorControl_RefNumRegistryGet.vi"("refnum name"="leftDrive") -> ("PhoenixMotorControlDevRef"=w1005:T5)  [unwired: 9 in, 1 out]
      n196 = call <vilib>:"CTRE_Phoenix_MotorControl_RefNumRegistryGet.vi"("refnum name"="rightDrive") -> ("PhoenixMotorControlDevRef"=w1004:T5)  [unwired: 9 in, 1 out]
      n197 = call <vilib>:"CTRE_Phoenix_MotorControl_RefNumRegistryGet.vi"("refnum name"="intake") -> ("PhoenixMotorControlDevRef"=w1002:T5)  [unwired: 9 in, 1 out]
      n198 = flat-sequence {
        tunnel: w1004 -> [w1061]
        tunnel: w1005 -> [w1062]
        tunnel: [w1060] -> w1052
        tunnel: [w1059] -> w1051
        tunnel: [w1058] -> w1050
        tunnel: w1002 -> [w1058]
        tunnel: w1001 -> [w1055]
        tunnel: [w1054] -> w1049
        tunnel: w1052 -> [w1071]
        tunnel: w1051 -> [w1070]
        tunnel: [w1067] -> w1048
        tunnel: w1050 -> [w1067]
        tunnel: [w1066] -> w1047
        tunnel: [w1065] -> w1046
        tunnel: w1049 -> [w1063]
        tunnel: [w1063] -> w1045
        tunnel: w1048 -> [w1079]
        tunnel: [w1079] -> w1044
        tunnel: w1047 -> [w1076]
        tunnel: w1046 -> [w1077]
        tunnel: [w1075] -> w1043
        tunnel: [w1074] -> w1042
        tunnel: w1045 -> [w1073]
        tunnel: [w1073] -> w1041
        tunnel: w1044 -> [w1088]
        tunnel: [w1088] -> w1040
        tunnel: w1043 -> [w1085]
        tunnel: w1042 -> [w1084]
        tunnel: [w1083] -> w1039
        tunnel: [w1082] -> w1038
        tunnel: w1041 -> [w1080]
        tunnel: [w1080] -> w1037
        tunnel: w1040 -> [w1096]
        tunnel: [w1096] -> w1036
        tunnel: w1039 -> [w1094]
        tunnel: w1038 -> [w1093]
        tunnel: [w1092] -> w1035
        tunnel: [w1091] -> w1034
        tunnel: w1037 -> [w1090]
        tunnel: [w1090] -> w1033
        tunnel: w1036 -> [w1104]
        tunnel: [w1103] -> w996
        tunnel: [w1099] -> w998
        tunnel: w1035 -> [w1099]
        tunnel: [w1098] -> w997
        tunnel: w1034 -> [w1098]
        tunnel: w1033 -> [w1097]
        tunnel: [w1097] -> w995
        tunnel: w998 -> [w1115]
        tunnel: w997 -> [w1114]
        tunnel: [w1113] -> w1032
        tunnel: [w1112] -> w1031
        tunnel: w996 -> [w1109]
        tunnel: [w1106] -> w1030
        tunnel: [w1105] -> w1029
        tunnel: w995 -> [w1105]
        tunnel: w1032 -> [w1127]
        tunnel: w1031 -> [w1126]
        tunnel: w1030 -> [w1119]
        tunnel: [w1124] -> w1028
        tunnel: [w1123] -> w1027
        tunnel: [w1122] -> w1026
        tunnel: w1029 -> [w1122]
        tunnel: [w1118] -> w999
        tunnel: [w1131] -> w1025
        tunnel: w1028 -> [w1131]
        tunnel: [w1130] -> w1024
        tunnel: w1027 -> [w1130]
        tunnel: [w1129] -> w1023
        tunnel: w1026 -> [w1129]
        tunnel: [w1128] -> w1022
        tunnel: w999 -> [w1128]
        tunnel: w1025 -> [w1149]
        tunnel: w1024 -> [w1148]
        tunnel: w1000 -> [w1137]
        tunnel: w1023 -> [w1146]
        tunnel: [w1139] -> w1021
        tunnel: [w1138] -> w1020
        tunnel: [w1137] -> w1019
        tunnel: [w1133] -> w1018
        tunnel: w1022 -> [w1134]
        tunnel: w1021 -> [w1160]
        tunnel: w1020 -> [w1159]
        tunnel: w1019 -> [w1153]
        tunnel: [w1158] -> w1017
        tunnel: [w1157] -> w1016
        tunnel: [w1153] -> w1015
        tunnel: [w1151] -> w1014
        tunnel: w1018 -> [w1151]
        tunnel: w1017 -> [w1171]
        tunnel: w1016 -> [w1170]
        tunnel: w1015 -> [w1163]
        tunnel: [w1165] -> w1013
        tunnel: [w1164] -> w1012
        tunnel: [w1163] -> w1011
        tunnel: [w1162] -> w1010
        tunnel: w1014 -> [w1162]
        tunnel: w1013 -> [w1178]
        tunnel: w1012 -> [w1179]
        tunnel: w1011 -> [w1175]
        tunnel: [w1172] -> w1009
        tunnel: w1010 -> [w1172]
        tunnel: w1009 -> [w1182]
        tunnel: [w1180] -> w1008
        tunnel: w1008 -> [w1185]
        frame #0 {
          # "Drive forward"
          n199 = call "auto_forward.vi"("timeout (ms)"=700.0, "distance (in)"=32.0 ("speed (decimal)"), "rightDrive"=w1061, "leftDrive"=w1062) -> ("rightDrive"=w1059:T5, "leftDrive"=w1060:T5)  [unwired: 6 in]
          n200 = call-poly <vilib>:"WPI_SolenoidSet.vi"("Value"=WPI_SolenoidValue."Reverse", "SolenoidDevRef"=w1055) -> ("SolenoidDevRef"=w1054:T2)  [unwired: 8 in, 1 out]
        }
        frame #1 {
          # "Turn towards exchange"
          n201 = call "auto_turn.vi"("direction"=enum16{"right", "left"}."left", "timeout (ms)"=1000.0, "angle"=90.0, "rightDrive"=w1070, "leftDrive"=w1071) -> ("rightDrive"=w1065:T5, "leftDrive"=w1066:T5)  [unwired: 5 in]
        }
        frame #2 {
          # "Drive into exchange area"
          n202 = call "auto_forward.vi"("timeout (ms)"=700.0, "distance (in)"=30.0 ("speed (decimal)"), "rightDrive"=w1077, "leftDrive"=w1076) -> ("rightDrive"=w1074:T5, "leftDrive"=w1075:T5)  [unwired: 6 in]
        }
        frame #3 {
          # "Face Exchange"
          n203 = call "auto_turn.vi"("direction"=enum16{"right", "left"}."left", "timeout (ms)"=1000.0, "angle"=90.0, "rightDrive"=w1084, "leftDrive"=w1085) -> ("rightDrive"=w1082:T5, "leftDrive"=w1083:T5)  [unwired: 5 in]
        }
        frame #4 {
          # "Drive up to exchange"
          n204 = call "auto_forward.vi"("timeout (ms)"=700.0, "distance (in)"=20.0 ("speed (decimal)"), "rightDrive"=w1093, "leftDrive"=w1094) -> ("rightDrive"=w1091:T5, "leftDrive"=w1092:T5)  [unwired: 6 in]
        }
        frame #5 {
          w1100 = T10 0 items=["PercentOutput"=0, "Position"=1, "Velocity"=2, "Current"=3, "Follower"=5, "MotionProfile"=6, "MotionMagic"=7, "MotionMagicArc"=8, "MotionProfileArc"=10, "Disabled"=15] ("Control Mode")
          # "Shoot cube in switch"
          n205 = call <vilib>:"CTRE_Phoenix_MotorControl_Set.vi"("Output"=-1.0, "Control Mode"=w1100, "PhoenixMotorControlDevRef"=w1104) -> ("PhoenixMotorControlDevRef"=w1103:T5)  [unwired: 7 in, 1 out]
          n206 = Wait (ms)(milliseconds to wait=u32 500) -> ()  [unwired: 1 out]
        }
        frame #6 {
          w1110 = T10 0 items=["PercentOutput"=0, "Position"=1, "Velocity"=2, "Current"=3, "Follower"=5, "MotionProfile"=6, "MotionMagic"=7, "MotionMagicArc"=8, "MotionProfileArc"=10, "Disabled"=15] ("Control Mode")
          # "Turn around to face the \ncube pyramid"
          n207 = call "auto_turn.vi"("direction"=enum16{"right", "left"}."left", "timeout (ms)"=1800.0, "angle"=166.0, "rightDrive"=w1114, "leftDrive"=w1115) -> ("rightDrive"=w1112:T5, "leftDrive"=w1113:T5)  [unwired: 5 in]
          n208 = call <vilib>:"CTRE_Phoenix_MotorControl_Set.vi"("Output"=0.0, "Control Mode"=w1110, "PhoenixMotorControlDevRef"=w1109) -> ("PhoenixMotorControlDevRef"=w1106:T5)  [unwired: 7 in, 1 out]
        }
        frame #7 {
          w1120 = T10 0 items=["PercentOutput"=0, "Position"=1, "Velocity"=2, "Current"=3, "Follower"=5, "MotionProfile"=6, "MotionMagic"=7, "MotionMagicArc"=8, "MotionProfileArc"=10, "Disabled"=15] ("Control Mode")
          # "Drive into pyramid\nwhile intaking"
          n209 = call "auto_forward.vi"("timeout (ms)"=1000.0, "distance (in)"=63.0, "rightDrive"=w1126, "leftDrive"=w1127) -> ("rightDrive"=w1123:T5, "leftDrive"=w1124:T5)  [unwired: 6 in]
          n210 = call <vilib>:"CTRE_Phoenix_MotorControl_Set.vi"("Output"=0.7, "Control Mode"=w1120, "PhoenixMotorControlDevRef"=w1119) -> ("PhoenixMotorControlDevRef"=w1118:T5)  [unwired: 7 in, 1 out]
        }
        frame #8 {
          # "Wait 2/5 of a second"
          n211 = Wait (ms)(milliseconds to wait=u32 400) -> ()  [unwired: 1 out]
        }
        frame #9 {
          w1135 = T10 0 items=["PercentOutput"=0, "Position"=1, "Velocity"=2, "Current"=3, "Follower"=5, "MotionProfile"=6, "MotionMagic"=7, "MotionMagicArc"=8, "MotionProfileArc"=10, "Disabled"=15] ("Control Mode")
          # "Turn towards hot side of \nswitch and lift intake"
          n212 = Select(t=enum16{"right", "left"}."right" ("direction"), s=w1137, f=enum16{"right", "left"}."left" ("direction")) -> (s? t:f=w1140:enum16{"right", "left"})
          n213 = Select(t=58.0, s=w1137, f=65.0) -> (s? t:f=w1141:dbl)
          n214 = call <vilib>:"CTRE_Phoenix_MotorControl_Set.vi"("Output"=0.0, "Control Mode"=w1135, "PhoenixMotorControlDevRef"=w1134) -> ("PhoenixMotorControlDevRef"=w1133:T5)  [unwired: 7 in, 1 out]
          n215 = call-poly <vilib>:"WPI_SolenoidSet.vi"("Value"=WPI_SolenoidValue."Forward", "SolenoidDevRef"=w1146) -> ()  [unwired: 8 in, 2 out]
          n216 = call "auto_turn.vi"("direction"=w1140, "timeout (ms)"=1500.0, "angle"=w1141, "rightDrive"=w1148, "leftDrive"=w1149) -> ("rightDrive"=w1138:T5, "leftDrive"=w1139:T5)  [unwired: 5 in]
        }
        frame #10 {
          # "Drive towards hot side of switch"
          n217 = Select(t=56.0, s=w1153, f=64.0) -> (s? t:f=w1156:dbl)
          n218 = call "auto_forward.vi"("timeout (ms)"=1500.0, "distance (in)"=w1156, "rightDrive"=w1159, "leftDrive"=w1160) -> ("rightDrive"=w1157:T5, "leftDrive"=w1158:T5)  [unwired: 6 in]
        }
        frame #11 {
          # "Turn and face switch"
          n219 = Select(t=67.0, s=w1163, f=0.0) -> (s? t:f=w1166:dbl)
          n220 = call "auto_turn.vi"("direction"=enum16{"right", "left"}."left", "timeout (ms)"=1000.0, "angle"=w1166, "rightDrive"=w1170, "leftDrive"=w1171) -> ("rightDrive"=w1164:T5, "leftDrive"=w1165:T5)  [unwired: 5 in]
        }
        frame #12 {
          # "Drive up to switch"
          n221 = Select(t=32.0, s=w1175, f=0.0) -> (s? t:f=w1174:dbl)
          n222 = call "auto_forward.vi"("timeout (ms)"=700.0, "distance (in)"=w1174, "rightDrive"=w1179, "leftDrive"=w1178) -> ()  [unwired: 6 in, 2 out]
        }
        frame #13 {
          w1183 = T10 0 items=["PercentOutput"=0, "Position"=1, "Velocity"=2, "Current"=3, "Follower"=5, "MotionProfile"=6, "MotionMagic"=7, "MotionMagicArc"=8, "MotionProfileArc"=10, "Disabled"=15] ("Control Mode")
          # "Shoot for one second"
          n223 = Wait (ms)(milliseconds to wait=u32 1000) -> ()  [unwired: 1 out]
          n224 = call <vilib>:"CTRE_Phoenix_MotorControl_Set.vi"("Output"=-0.5, "Control Mode"=w1183, "PhoenixMotorControlDevRef"=w1182) -> ("PhoenixMotorControlDevRef"=w1180:T5)  [unwired: 7 in, 1 out]
        }
        frame #14 {
          w1186 = T10 0 items=["PercentOutput"=0, "Position"=1, "Velocity"=2, "Current"=3, "Follower"=5, "MotionProfile"=6, "MotionMagic"=7, "MotionMagicArc"=8, "MotionProfileArc"=10, "Disabled"=15] ("Control Mode")
          # "Stop shooting"
          n225 = call <vilib>:"CTRE_Phoenix_MotorControl_Set.vi"("Output"=0.0, "Control Mode"=w1186, "PhoenixMotorControlDevRef"=w1185) -> ()  [unwired: 7 in, 2 out]
        }
      }
    }
    frame "hot_from_middle_diagonal" {
      n226 = call <vilib>:"CTRE_Phoenix_MotorControl_RefNumRegistryGet.vi"("refnum name"="leftDrive") -> ("PhoenixMotorControlDevRef"=w1211:T5)  [unwired: 9 in, 1 out]
      n227 = call <vilib>:"CTRE_Phoenix_MotorControl_RefNumRegistryGet.vi"("refnum name"="rightDrive") -> ("PhoenixMotorControlDevRef"=w1210:T5)  [unwired: 9 in, 1 out]
      n228 = call <vilib>:"CTRE_Phoenix_MotorControl_RefNumRegistryGet.vi"("refnum name"="intake") -> ("PhoenixMotorControlDevRef"=w1200:T5)  [unwired: 9 in, 1 out]
      n229 = flat-sequence {
        tunnel: w1211 -> [w1219]
        tunnel: w1210 -> [w1218]
        tunnel: [w1215] -> w1207
        tunnel: [w1214] -> w1206
        tunnel: w1205 -> [w1213]
        tunnel: [w1213] -> w1204
        tunnel: [w1212] -> w1201
        tunnel: w1200 -> [w1212]
        tunnel: w1207 -> [w1230]
        tunnel: w1206 -> [w1229]
        tunnel: w1204 -> [w1220]
        tunnel: [w1223] -> w1203
        tunnel: [w1222] -> w1202
        tunnel: w1201 -> [w1221]
        tunnel: [w1221] -> w1199
        tunnel: [w1220] -> w1192
        tunnel: w1203 -> [w1238]
        tunnel: w1202 -> [w1237]
        tunnel: [w1234] -> w1196
        tunnel: w1199 -> [w1234]
        tunnel: [w1233] -> w1195
        tunnel: [w1232] -> w1194
        tunnel: [w1231] -> w1193
        tunnel: w1192 -> [w1231]
        tunnel: w1196 -> [w1249]
        tunnel: [w1249] -> w1191
        tunnel: w1195 -> [w1248]
        tunnel: w1194 -> [w1247]
        tunnel: w1193 -> [w1245]
        tunnel: [w1240] -> w1190
        tunnel: [w1239] -> w1189
        tunnel: w1191 -> [w1254]
        tunnel: [w1254] -> w1188
        tunnel: w1190 -> [w1253]
        tunnel: w1189 -> [w1252]
        tunnel: w1188 -> [w1259]
        tunnel: [w1255] -> w1197
        tunnel: w1197 -> [w1262]
        frame #0 {
          n230 = call "auto_forward.vi"("timeout (ms)"=1250.0, "distance (in)"=30.0, "rightDrive"=w1218, "leftDrive"=w1219) -> ("rightDrive"=w1214:T5, "leftDrive"=w1215:T5)  [unwired: 6 in]
        }
        frame #1 {
          n231 = Select(t=enum16{"right", "left"}."right" ("direction"), s=w1220, f=enum16{"right", "left"}."left" ("direction")) -> (s? t:f=w1226:enum16{"right", "left"})
          n232 = call "auto_turn.vi"("direction"=w1226, "timeout (ms)"=1200.0, "angle"=45.0, "rightDrive"=w1229, "leftDrive"=w1230) -> ("rightDrive"=w1222:T5, "leftDrive"=w1223:T5)  [unwired: 5 in]
        }
        frame #2 {
          n233 = call "auto_forward.vi"("timeout (ms)"=1500.0, "distance (in)"=72.0, "rightDrive"=w1237, "leftDrive"=w1238) -> ("rightDrive"=w1232:T5, "leftDrive"=w1233:T5)  [unwired: 6 in]
        }
        frame #3 {
          n234 = Select(t=enum16{"right", "left"}."left" ("direction"), s=w1245, f=enum16{"right", "left"}."right" ("direction")) -> (s? t:f=w1242:enum16{"right", "left"})
          n235 = call "auto_turn.vi"("direction"=w1242, "timeout (ms)"=1200.0, "angle"=45.0, "rightDrive"=w1247, "leftDrive"=w1248) -> ("rightDrive"=w1239:T5, "leftDrive"=w1240:T5)  [unwired: 5 in]
        }
        frame #4 {
          n236 = call "auto_forward.vi"("timeout (ms)"=700.0, "distance (in)"=25.0, "rightDrive"=w1252, "leftDrive"=w1253) -> ()  [unwired: 6 in, 2 out]
        }
        frame #5 {
          w1258 = T10 0 items=["PercentOutput"=0, "Position"=1, "Velocity"=2, "Current"=3, "Follower"=5, "MotionProfile"=6, "MotionMagic"=7, "MotionMagicArc"=8, "MotionProfileArc"=10, "Disabled"=15] ("Control Mode")
          n237 = call <vilib>:"CTRE_Phoenix_MotorControl_Set.vi"("Output"=-0.8, "Control Mode"=w1258, "PhoenixMotorControlDevRef"=w1259) -> ("PhoenixMotorControlDevRef"=w1255:T5)  [unwired: 7 in, 1 out]
          n238 = Wait (ms)(milliseconds to wait=u32 2500) -> ()  [unwired: 1 out]
        }
        frame #6 {
          w1261 = T10 0 items=["PercentOutput"=0, "Position"=1, "Velocity"=2, "Current"=3, "Follower"=5, "MotionProfile"=6, "MotionMagic"=7, "MotionMagicArc"=8, "MotionProfileArc"=10, "Disabled"=15] ("Control Mode")
          n239 = call <vilib>:"CTRE_Phoenix_MotorControl_Set.vi"("Output"=0.0, "Control Mode"=w1261, "PhoenixMotorControlDevRef"=w1262) -> ()  [unwired: 7 in, 2 out]
        }
      }
    }
    frame "yet to be named" {
      n240 = flat-sequence {
        frame #0 {
        }
      }
    }
    frame "If_hot_1_else_baseline" {
      # "True means cold"
      n241 = Not Exclusive Or(1:w1266, 2:w1265) -> (0:w1269:bool)
      n242 = call <vilib>:"CTRE_Phoenix_MotorControl_RefNumRegistryGet.vi"("refnum name"="rightDrive") -> ("PhoenixMotorControlDevRef"=w1272:T5)  [unwired: 9 in, 1 out]
      n243 = call <vilib>:"CTRE_Phoenix_MotorControl_RefNumRegistryGet.vi"("refnum name"="leftDrive") -> ("PhoenixMotorControlDevRef"=w1273:T5)  [unwired: 9 in, 1 out]
      n244 = call <vilib>:"CTRE_Phoenix_MotorControl_RefNumRegistryGet.vi"("refnum name"="intake") -> ("PhoenixMotorControlDevRef"=w1271:T5)  [unwired: 9 in, 1 out]
      n245 = flat-sequence {
        tunnel: w1273 -> [w1300]
        tunnel: w1272 -> [w1299]
        tunnel: w1269 -> [w1296]
        tunnel: [w1298] -> w1291
        tunnel: [w1297] -> w1290
        tunnel: [w1296] -> w1289
        tunnel: w1271 -> [w1295]
        tunnel: [w1295] -> w1288
        tunnel: [w1294] -> w1287
        tunnel: w1264 -> [w1294]
        tunnel: [w1293] -> w1286
        tunnel: w1266 -> [w1293]
        tunnel: w1291 -> [w1318]
        tunnel: w1290 -> [w1317]
        tunnel: w1289 -> [w1316]
        tunnel: [w1316] -> w1285
        tunnel: [w1312] -> w1284
        tunnel: [w1311] -> w1283
        tunnel: w1288 -> [w1310]
        tunnel: [w1310] -> w1282
        tunnel: w1287 -> [w1309]
        tunnel: [w1309] -> w1281
        tunnel: w1286 -> [w1305]
        tunnel: [w1305] -> w1280
        tunnel: w1285 -> [w1322]
        tunnel: w1284 -> [w1327]
        tunnel: w1283 -> [w1326]
        tunnel: w1282 -> [w1325]
        tunnel: [w1325] -> w1279
        tunnel: [w1324] -> w1278
        tunnel: [w1323] -> w1277
        tunnel: [w1322] -> w1276
        tunnel: [w1321] -> w1275
        tunnel: w1281 -> [w1321]
        tunnel: [w1319] -> w1274
        tunnel: w1280 -> [w1319]
        tunnel: w1279 -> [w1338]
        tunnel: w1278 -> [_]
        tunnel: w1277 -> [_]
        tunnel: w1276 -> [w1335]
        tunnel: w1275 -> [_]
        tunnel: w1274 -> [_]
        tunnel: [w1331] -> w1263
        tunnel: w1263 -> [w1341]
        frame #0 {
          # "If starting on the cold side\ncross the baseline. If the hot\nside drive up to the side of the\nswitch"
          n246 = Select(t=152.75, s=w1296, f=100.0) -> (s? t:f=w1301:dbl)
          n247 = call "auto_forward.vi"("timeout (ms)"=2000.0, "distance (in)"=w1301, "rightDrive"=w1299, "leftDrive"=w1300) -> ("rightDrive"=w1297:T5, "leftDrive"=w1298:T5)  [unwired: 6 in]
        }
        frame #1 {
          # "Turn and face the switch"
          n248 = Select(t=enum16{"right", "left"}."left" ("direction"), s=w1305, f=enum16{"right", "left"}."right" ("direction")) -> (s? t:f=w1308:enum16{"right", "left"})
          n249 = Select(t=90.0, s=w1316, f=0.0) -> (s? t:f=w1313:dbl)
          n250 = call "auto_turn.vi"("direction"=w1308, "timeout (ms)"=3000.0, "angle"=w1313, "rightDrive"=w1317, "leftDrive"=w1318) -> ("rightDrive"=w1311:T5, "leftDrive"=w1312:T5)  [unwired: 5 in]
        }
        frame #2 {
          # "Drive up to the switch"
          n251 = Select(t=40.0, s=w1322, f=0.0) -> (s? t:f=w1328:dbl)
          n252 = call "auto_forward.vi"("timeout (ms)"=1000.0, "distance (in)"=w1328, "rightDrive"=w1326, "leftDrive"=w1327) -> ("rightDrive"=w1323:T5, "leftDrive"=w1324:T5)  [unwired: 6 in]
        }
        frame #3 {
          w1337 = T10 0 items=["PercentOutput"=0, "Position"=1, "Velocity"=2, "Current"=3, "Follower"=5, "MotionProfile"=6, "MotionMagic"=7, "MotionMagicArc"=8, "MotionProfileArc"=10, "Disabled"=15] ("Control Mode")
          # "Shoot a cube into the switch for\n1 second"
          n253 = Select(t=-0.8, s=w1335, f=0.0) -> (s? t:f=w1332:dbl)
          n254 = Wait (ms)(milliseconds to wait=u32 1000) -> ()  [unwired: 1 out]
          n255 = call <vilib>:"CTRE_Phoenix_MotorControl_Set.vi"("Output"=w1332, "Control Mode"=w1337, "PhoenixMotorControlDevRef"=w1338) -> ("PhoenixMotorControlDevRef"=w1331:T5)  [unwired: 7 in, 1 out]
        }
        frame #4 {
          w1340 = T10 0 items=["PercentOutput"=0, "Position"=1, "Velocity"=2, "Current"=3, "Follower"=5, "MotionProfile"=6, "MotionMagic"=7, "MotionMagicArc"=8, "MotionProfileArc"=10, "Disabled"=15] ("Control Mode")
          # "Stop shooter"
          n256 = call <vilib>:"CTRE_Phoenix_MotorControl_Set.vi"("Output"=0.0, "Control Mode"=w1340, "PhoenixMotorControlDevRef"=w1341) -> ()  [unwired: 7 in, 2 out]
        }
      }
    }
    frame "hot_2_from_middle" {
      n257 = call <vilib>:"CTRE_Phoenix_MotorControl_RefNumRegistryGet.vi"("refnum name"="leftDrive") -> ("PhoenixMotorControlDevRef"=w1393:T5)  [unwired: 9 in, 1 out]
      n258 = call <vilib>:"CTRE_Phoenix_MotorControl_RefNumRegistryGet.vi"("refnum name"="rightDrive") -> ("PhoenixMotorControlDevRef"=w1392:T5)  [unwired: 9 in, 1 out]
      n259 = call <vilib>:"CTRE_Phoenix_MotorControl_RefNumRegistryGet.vi"("refnum name"="intake") -> ("PhoenixMotorControlDevRef"=w1391:T5)  [unwired: 9 in, 1 out]
      n260 = flat-sequence {
        tunnel: w1393 -> [w1423]
        tunnel: w1392 -> [w1422]
        tunnel: [w1420] -> w1413
        tunnel: [w1417] -> w1412
        tunnel: w1390 -> [w1419]
        tunnel: [w1419] -> w1411
        tunnel: [w1418] -> w1410
        tunnel: w1391 -> [w1418]
        tunnel: w1375 -> [w1414]
        tunnel: [w1414] -> w1370
        tunnel: w1413 -> [w1435]
        tunnel: w1412 -> [w1434]
        tunnel: w1411 -> [w1427]
        tunnel: [w1429] -> w1409
        tunnel: [w1428] -> w1408
        tunnel: [w1427] -> w1407
        tunnel: [w1426] -> w1406
        tunnel: w1410 -> [w1426]
        tunnel: [w1424] -> w1371
        tunnel: w1370 -> [w1424]
        tunnel: w1409 -> [w1446]
        tunnel: w1408 -> [w1445]
        tunnel: [w1444] -> w1405
        tunnel: [w1443] -> w1404
        tunnel: w1407 -> [w1436]
        tunnel: [w1436] -> w1403
        tunnel: [w1442] -> w1402
        tunnel: w1406 -> [w1442]
        tunnel: [w1440] -> w1372
        tunnel: w1371 -> [w1440]
        tunnel: [w1436] -> w1346
        tunnel: w1405 -> [w1457]
        tunnel: w1404 -> [w1456]
        tunnel: w1403 -> [w1451]
        tunnel: [w1455] -> w1401
        tunnel: [w1454] -> w1400
        tunnel: [w1453] -> w1399
        tunnel: w1402 -> [w1453]
        tunnel: [w1451] -> w1380
        tunnel: [w1450] -> w1373
        tunnel: w1372 -> [w1450]
        tunnel: w1346 -> [w1448]
        tunnel: [w1448] -> w1342
        tunnel: w1401 -> [w1472]
        tunnel: w1400 -> [w1471]
        tunnel: [w1470] -> w1398
        tunnel: w1399 -> [w1470]
        tunnel: [w1468] -> w1388
        tunnel: [w1467] -> w1386
        tunnel: [w1463] -> w1381
        tunnel: w1380 -> [w1463]
        tunnel: [w1466] -> w1374
        tunnel: w1373 -> [w1466]
        tunnel: [w1461] -> w1343
        tunnel: w1342 -> [w1461]
        tunnel: w1398 -> [w1483]
        tunnel: [w1480] -> w1397
        tunnel: [w1478] -> w1389
        tunnel: w1388 -> [w1478]
        tunnel: [w1477] -> w1387
        tunnel: w1386 -> [w1477]
        tunnel: [w1476] -> w1382
        tunnel: w1381 -> [w1476]
        tunnel: w1374 -> [w1475]
        tunnel: [w1475] -> w1369
        tunnel: [w1474] -> w1344
        tunnel: w1343 -> [w1474]
        tunnel: w1397 -> [w1497]
        tunnel: w1389 -> [w1496]
        tunnel: w1387 -> [w1495]
        tunnel: [w1491] -> w1385
        tunnel: [w1490] -> w1384
        tunnel: [w1489] -> w1383
        tunnel: w1382 -> [w1489]
        tunnel: [w1488] -> w1376
        tunnel: w1369 -> [w1487]
        tunnel: [w1485] -> w1367
        tunnel: [w1484] -> w1345
        tunnel: w1344 -> [w1484]
        tunnel: w1385 -> [w1514]
        tunnel: w1384 -> [w1513]
        tunnel: w1383 -> [w1504]
        tunnel: [w1509] -> w1379
        tunnel: [w1508] -> w1378
        tunnel: [w1506] -> w1377
        tunnel: w1376 -> [w1506]
        tunnel: [w1505] -> w1368
        tunnel: w1367 -> [w1505]
        tunnel: [w1504] -> w1364
        tunnel: w1345 -> [w1500]
        tunnel: w1379 -> [w1526]
        tunnel: w1378 -> [w1525]
        tunnel: w1377 -> [w1522]
        tunnel: [w1519] -> w1357
        tunnel: [w1518] -> w1355
        tunnel: [w1517] -> w1353
        tunnel: w1368 -> [w1517]
        tunnel: [w1516] -> w1351
        tunnel: w1364 -> [w1516]
        tunnel: [w1515] -> w1349
        tunnel: w1357 -> [w1532]
        tunnel: [w1532] -> w1356
        tunnel: w1355 -> [w1531]
        tunnel: [w1531] -> w1354
        tunnel: w1353 -> [w1530]
        tunnel: [w1530] -> w1352
        tunnel: w1351 -> [w1529]
        tunnel: [w1529] -> w1350
        tunnel: w1349 -> [w1528]
        tunnel: [w1528] -> w1348
        tunnel: w1356 -> [w1546]
        tunnel: w1354 -> [w1545]
        tunnel: w1352 -> [w1541]
        tunnel: [w1539] -> w1366
        tunnel: [w1538] -> w1365
        tunnel: w1350 -> [w1538]
        tunnel: [w1537] -> w1363
        tunnel: [w1533] -> w1358
        tunnel: w1348 -> [w1534]
        tunnel: w1366 -> [w1557]
        tunnel: w1365 -> [w1556]
        tunnel: w1363 -> [w1552]
        tunnel: [w1550] -> w1362
        tunnel: [w1549] -> w1361
        tunnel: [w1547] -> w1359
        tunnel: w1358 -> [w1547]
        tunnel: w1362 -> [w1562]
        tunnel: w1361 -> [w1561]
        tunnel: [w1558] -> w1360
        tunnel: w1359 -> [w1558]
        tunnel: w1360 -> [w1567]
        tunnel: [w1563] -> w1347
        tunnel: w1347 -> [w1569]
        frame #0 {
          # "Drive forward towards\npyramid"
          n261 = call "auto_forward.vi"("reverse?"=FALSE, "timeout (ms)"=1250.0, "distance (in)"=30.0, "rightDrive"=w1422, "leftDrive"=w1423) -> ("rightDrive"=w1417:T5, "leftDrive"=w1420:T5)  [unwired: 5 in]
        }
        frame #1 {
          # "Turn left or right \ndepending on hot side"
          n262 = Select(t=enum16{"right", "left"}."right" ("direction"), s=w1427, f=enum16{"right", "left"}."left" ("direction")) -> (s? t:f=w1430:enum16{"right", "left"})
          n263 = call "auto_turn.vi"("direction"=w1430, "timeout (ms)"=1200.0, "angle"=45.0, "rightDrive"=w1434, "leftDrive"=w1435) -> ("rightDrive"=w1428:T5, "leftDrive"=w1429:T5)  [unwired: 5 in]
        }
        frame #2 {
          # "Drive forward to\nget around pyramid"
          n264 = Select(t=72.0 ("distance (in)"), s=w1436, f=90.0) -> (s? t:f=w1438:dbl)
          n265 = call "auto_forward.vi"("reverse?"=FALSE, "timeout (ms)"=1500.0, "distance (in)"=w1438, "rightDrive"=w1445, "leftDrive"=w1446) -> ("rightDrive"=w1443:T5, "leftDrive"=w1444:T5)  [unwired: 5 in]
        }
        frame #3 {
          # "Turn to face the switch"
          n266 = Select(t=enum16{"right", "left"}."left" ("direction"), s=w1451, f=enum16{"right", "left"}."right" ("direction")) -> (s? t:f=w1458:enum16{"right", "left"})
          n267 = call "auto_turn.vi"("direction"=w1458, "timeout (ms)"=1200.0, "angle"=45.0, "rightDrive"=w1456, "leftDrive"=w1457) -> ("rightDrive"=w1454:T5, "leftDrive"=w1455:T5)  [unwired: 5 in]
        }
        frame #4 {
          # "Drive up to the\nswitch"
          n268 = Select(t=33.0 ("distance (in)"), s=w1463, f=22.0) -> (s? t:f=w1462:dbl)
          n269 = call "auto_forward.vi"("reverse?"=FALSE, "timeout (ms)"=800.0, "distance (in)"=w1462, "rightDrive"=w1471, "leftDrive"=w1472) -> ("rightDrive"=w1467:T5, "leftDrive"=w1468:T5)  [unwired: 5 in]
        }
        frame #5 {
          w1482 = T10 0 items=["PercentOutput"=0, "Position"=1, "Velocity"=2, "Current"=3, "Follower"=5, "MotionProfile"=6, "MotionMagic"=7, "MotionMagicArc"=8, "MotionProfileArc"=10, "Disabled"=15] ("Control Mode")
          # "Shoot cube for \n0.75 seconds"
          n270 = Wait (ms)(milliseconds to wait=u32 500) -> ()  [unwired: 1 out]
          n271 = call <vilib>:"CTRE_Phoenix_MotorControl_Set.vi"("Output"=-0.7, "Control Mode"=w1482, "PhoenixMotorControlDevRef"=w1483) -> ("PhoenixMotorControlDevRef"=w1480:T5)  [unwired: 7 in, 1 out]
        }
        frame #6 {
          w1499 = T10 0 items=["PercentOutput"=0, "Position"=1, "Velocity"=2, "Current"=3, "Follower"=5, "MotionProfile"=6, "MotionMagic"=7, "MotionMagicArc"=8, "MotionProfileArc"=10, "Disabled"=15] ("Control Mode")
          # "Set shooter output\nback to 0"
          n272 = call "auto_forward.vi"("reverse?"=TRUE, "timeout (ms)"=1500.0, "distance (in)"=70.0, "rightDrive"=w1495, "leftDrive"=w1496) -> ("rightDrive"=w1490:T5, "leftDrive"=w1491:T5)  [unwired: 5 in]
          n273 = call-poly <vilib>:"WPI_SolenoidSet.vi"("Value"=WPI_SolenoidValue."Reverse", "SolenoidDevRef"=w1487) -> ("SolenoidDevRef"=w1485:T2)  [unwired: 8 in, 1 out]
          n274 = call <vilib>:"CTRE_Phoenix_MotorControl_Set.vi"("Output"=0.0, "Control Mode"=w1499, "PhoenixMotorControlDevRef"=w1497) -> ("PhoenixMotorControlDevRef"=w1488:T5)  [unwired: 7 in, 1 out]
        }
        frame #7 {
          n275 = Select(t=49.0 ("angle"), s=w1500, f=49.0) -> (s? t:f=w1501:dbl)
          n276 = Select(t=enum16{"right", "left"}."left" ("direction"), s=w1504, f=enum16{"right", "left"}."right" ("direction")) -> (s? t:f=w1510:enum16{"right", "left"})
          n277 = call "auto_turn.vi"("direction"=w1510, "timeout (ms)"=1000.0, "angle"=w1501, "rightDrive"=w1513, "leftDrive"=w1514) -> ("rightDrive"=w1508:T5, "leftDrive"=w1509:T5)  [unwired: 5 in]
        }
        frame #8 {
          w1521 = T10 0 items=["PercentOutput"=0, "Position"=1, "Velocity"=2, "Current"=3, "Follower"=5, "MotionProfile"=6, "MotionMagic"=7, "MotionMagicArc"=8, "MotionProfileArc"=10, "Disabled"=15] ("Control Mode")
          n278 = call <vilib>:"CTRE_Phoenix_MotorControl_Set.vi"("Output"=0.75, "Control Mode"=w1521, "PhoenixMotorControlDevRef"=w1522) -> ("PhoenixMotorControlDevRef"=w1515:T5)  [unwired: 7 in, 1 out]
          n279 = call "auto_forward.vi"("timeout (ms)"=1500.0, "distance (in)"=55.0, "rightDrive"=w1525, "leftDrive"=w1526) -> ("rightDrive"=w1518:T5, "leftDrive"=w1519:T5)  [unwired: 6 in]
        }
        frame #9 {
          n280 = Wait (ms)(milliseconds to wait=u32 300) -> ()  [unwired: 1 out]
        }
        frame #10 {
          w1536 = T10 0 items=["PercentOutput"=0, "Position"=1, "Velocity"=2, "Current"=3, "Follower"=5, "MotionProfile"=6, "MotionMagic"=7, "MotionMagicArc"=8, "MotionProfileArc"=10, "Disabled"=15] ("Control Mode")
          n281 = call-poly <vilib>:"WPI_SolenoidSet.vi"("Value"=WPI_SolenoidValue."Forward", "SolenoidDevRef"=w1541) -> ()  [unwired: 8 in, 2 out]
          n282 = call "auto_forward.vi"("reverse?"=TRUE, "timeout (ms)"=1250.0, "distance (in)"=45.0, "rightDrive"=w1545, "leftDrive"=w1546) -> ("rightDrive"=w1537:T5, "leftDrive"=w1539:T5)  [unwired: 5 in]
          n283 = call <vilib>:"CTRE_Phoenix_MotorControl_Set.vi"("Output"=0.0, "Control Mode"=w1536, "PhoenixMotorControlDevRef"=w1534) -> ("PhoenixMotorControlDevRef"=w1533:T5)  [unwired: 7 in, 1 out]
        }
        frame #11 {
          n284 = Select(t=enum16{"right", "left"}."right" ("direction"), s=w1556, f=enum16{"right", "left"}."left" ("direction")) -> (s? t:f=w1553:enum16{"right", "left"})
          n285 = call "auto_turn.vi"("direction"=w1553, "timeout (ms)"=1000.0, "angle"=49.0, "rightDrive"=w1552, "leftDrive"=w1557) -> ("rightDrive"=w1549:T5, "leftDrive"=w1550:T5)  [unwired: 5 in]
        }
        frame #12 {
          n286 = call "auto_forward.vi"("timeout (ms)"=1200.0, "distance (in)"=68.0, "rightDrive"=w1561, "leftDrive"=w1562) -> ()  [unwired: 6 in, 2 out]
        }
        frame #13 {
          w1565 = T10 0 items=["PercentOutput"=0, "Position"=1, "Velocity"=2, "Current"=3, "Follower"=5, "MotionProfile"=6, "MotionMagic"=7, "MotionMagicArc"=8, "MotionProfileArc"=10, "Disabled"=15] ("Control Mode")
          n287 = call <vilib>:"CTRE_Phoenix_MotorControl_Set.vi"("Output"=-0.7, "Control Mode"=w1565, "PhoenixMotorControlDevRef"=w1567) -> ("PhoenixMotorControlDevRef"=w1563:T5)  [unwired: 7 in, 1 out]
          n288 = Wait (ms)(milliseconds to wait=u32 1500) -> ()  [unwired: 1 out]
        }
        frame #14 {
          w1568 = T10 0 items=["PercentOutput"=0, "Position"=1, "Velocity"=2, "Current"=3, "Follower"=5, "MotionProfile"=6, "MotionMagic"=7, "MotionMagicArc"=8, "MotionProfileArc"=10, "Disabled"=15] ("Control Mode")
          n289 = call <vilib>:"CTRE_Phoenix_MotorControl_Set.vi"("Output"=0.0, "Control Mode"=w1568, "PhoenixMotorControlDevRef"=w1569) -> ()  [unwired: 7 in, 2 out]
        }
      }
    }
  }
